vi "User_Login.vi"() -> ()   [LabVIEW 2019]
uses:
  <vilib>/Utility/file.llb/Read Delimited Spreadsheet (string).vi
  <vilib>/Utility/file.llb/Write Delimited Spreadsheet (string).vi
  <vilib>/Utility/file.llb/Write Delimited Spreadsheet (I64).vi
  <vilib>/numeric/Random Number (Range) U64.vi
panel:
  out "测试":bool
  in  "数组":u64[](array[numeric])
  in  "亮灯次数":i32=1
  in  "是否开始计时？":bool
  out "分数":i32
  out "难度":string="困难"
  out "闪烁间隔":i32=727
  out "超时时间":i32=500
  out "User name out":string
  out "时间到":bool
  out "字符串":string
  in  "选项卡控件":T1(tab)
  in  "密码":string
  in  "账号":string
  in  "登录界面_修改密码":bool
  in  "登陆界面_注册":bool
  in  "登录界面_登录":bool
  in  "登录界面_退出":bool
  in  "主界面_TOP10":bool
  in  "主界面_返回":bool
  in  "主界面_进入游戏":bool
  in  "主界面_游戏规则":bool
  in  "注册簇":T2
  in  "用户注册_注册":bool
  in  "用户注册_返回":bool
  in  "修改密码簇":T3
  in  "修改密码_返回":bool
  in  "修改密码_修改":bool
  in  "TOP10_返回":bool
  in  "游戏规则_返回":bool
  in  "读档":bool
  in  "存档":bool
  out "难度：分数":string
  out "倒计时":i32(slide) scale=-1.0..3635.0
  in  "User name in":string
  in  "结束":bool
  out "上":bool
  out "左":bool
  out "右":bool
  out "下":bool
  in  "OK":bool
  # "游戏开始时，第一次亮一\n个灯，然后我们需要点击一次已 \n，第二次会亮两个灯，包括第一\n次的灯，第三次亮三个，每次增\n加一个灯，你都需要按顺序点击\n，或者使用键盘的↑↓←→操作"
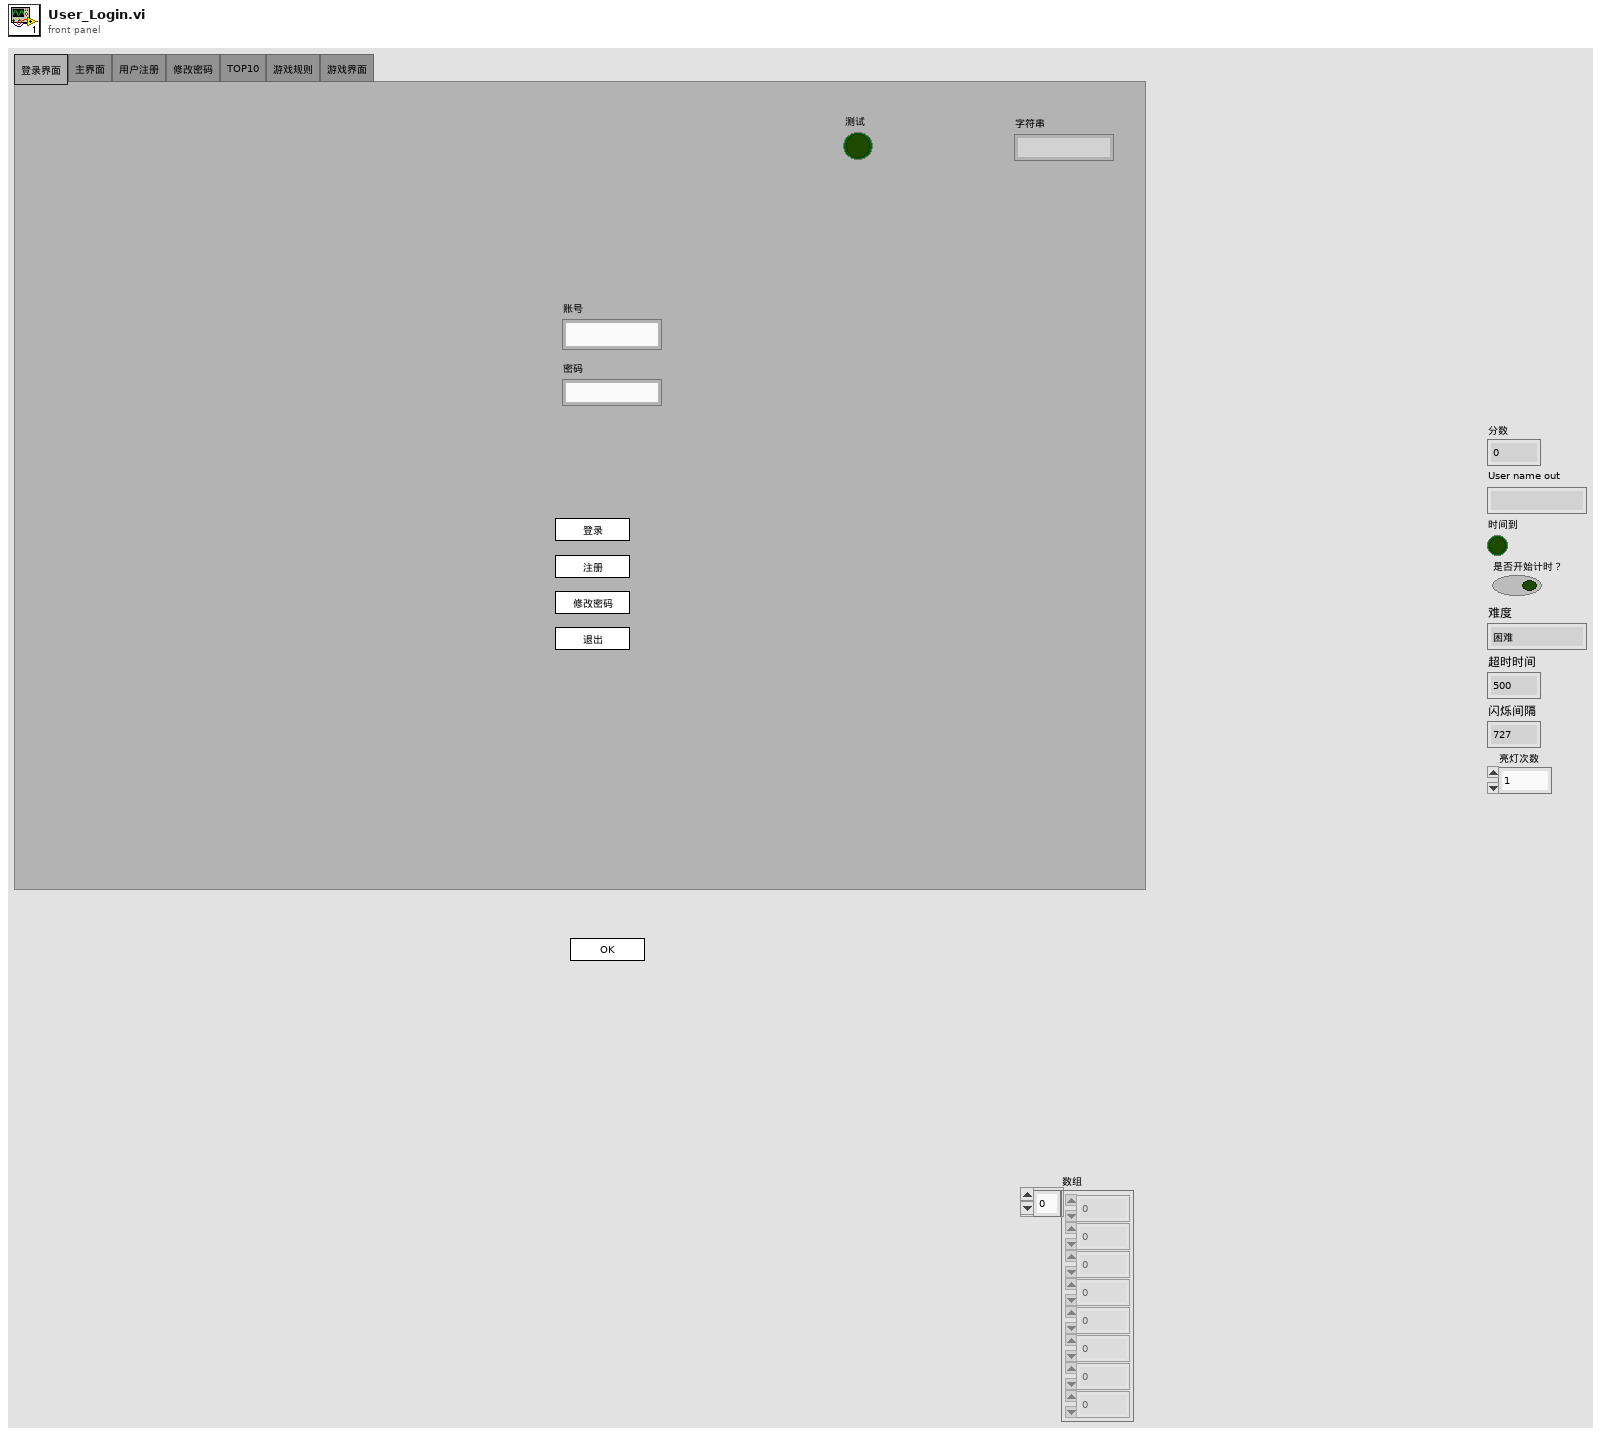
[diagram p1: front panel]
types:
  T1 = enum32{"登录界面", "主界面", "用户注册", "修改密码", "TOP10", "游戏规则", "游戏界面"}
  T2 = cluster{"注册账户":string, "注册密码":string, "确认密码":string}
  T3 = cluster{"账号":string, "旧密码":string, "新密码":string, "确认密码":string}
  T4 = typedef "选项卡枚举.ctl" = enum32{"登录界面", "主界面", "用户注册", "修改密码", "TOP10", "游戏规则", "游戏界面"}
  T5 = enum32{"Invalid", "Standard", "Closed", "Hidden", "Minimized", "Maximized"}
  T6 = enum32{"invalid app kind", "Development System", "Run Time System", "Student Edition", "Embedded LabVIEW", "Evaluation", "Custom"}
  T7 = typedef "按键枚举.ctl" = enum16{"读档", "存档", "按错", "退出", "黄", "红", "蓝", "绿"}
  T8 = cluster{"Core":cluster{"Current VI Reference":refnum<vi>, "Close Panel on Exit?":bool}, "Your Boolean data":bool, "注册账户":string, "注册密码":string, "修改密码_新密码":string, "修改密码_账户":string, "用户名":string, "难度_保存":string, "亮灯次数_保存":i32, "超时时间_保存":i32, "闪烁间隔_保存":i32, "积分_保存":i32}
  T9 = cluster{"Current VI Reference":refnum<vi>, "Close Panel on Exit?":bool}
  T10 = enum16{"Left Button", "Center Button", "Right Button", "Window Close"}
  T11 = typedef "eventvkey.ctl" = enum16{"ASCII", "Enter", "Return", "Shift", "Ctrl", "Alt", "Cmd", "Opt", "Caps", "NumLock", "Clear", "Break", "Up", "Down", "Left", "Right", "Insert", "Delete", "Home", "End", "PageUp", "PageDown", "Escape", "Help", "Pause", "ScrollLock", "F1", "F2", "F3", "F4", "F5", "F6", "F7", "F8", "F9", "F10", "F11", "F12", "F13", "F14", "F15", "F16", "F17", "F18", "F19", "F20", "F21", "F22", "F23", "F24", "Play", "VolumeUp", "VolumeDown", "Mute", "Two Byte Char"}
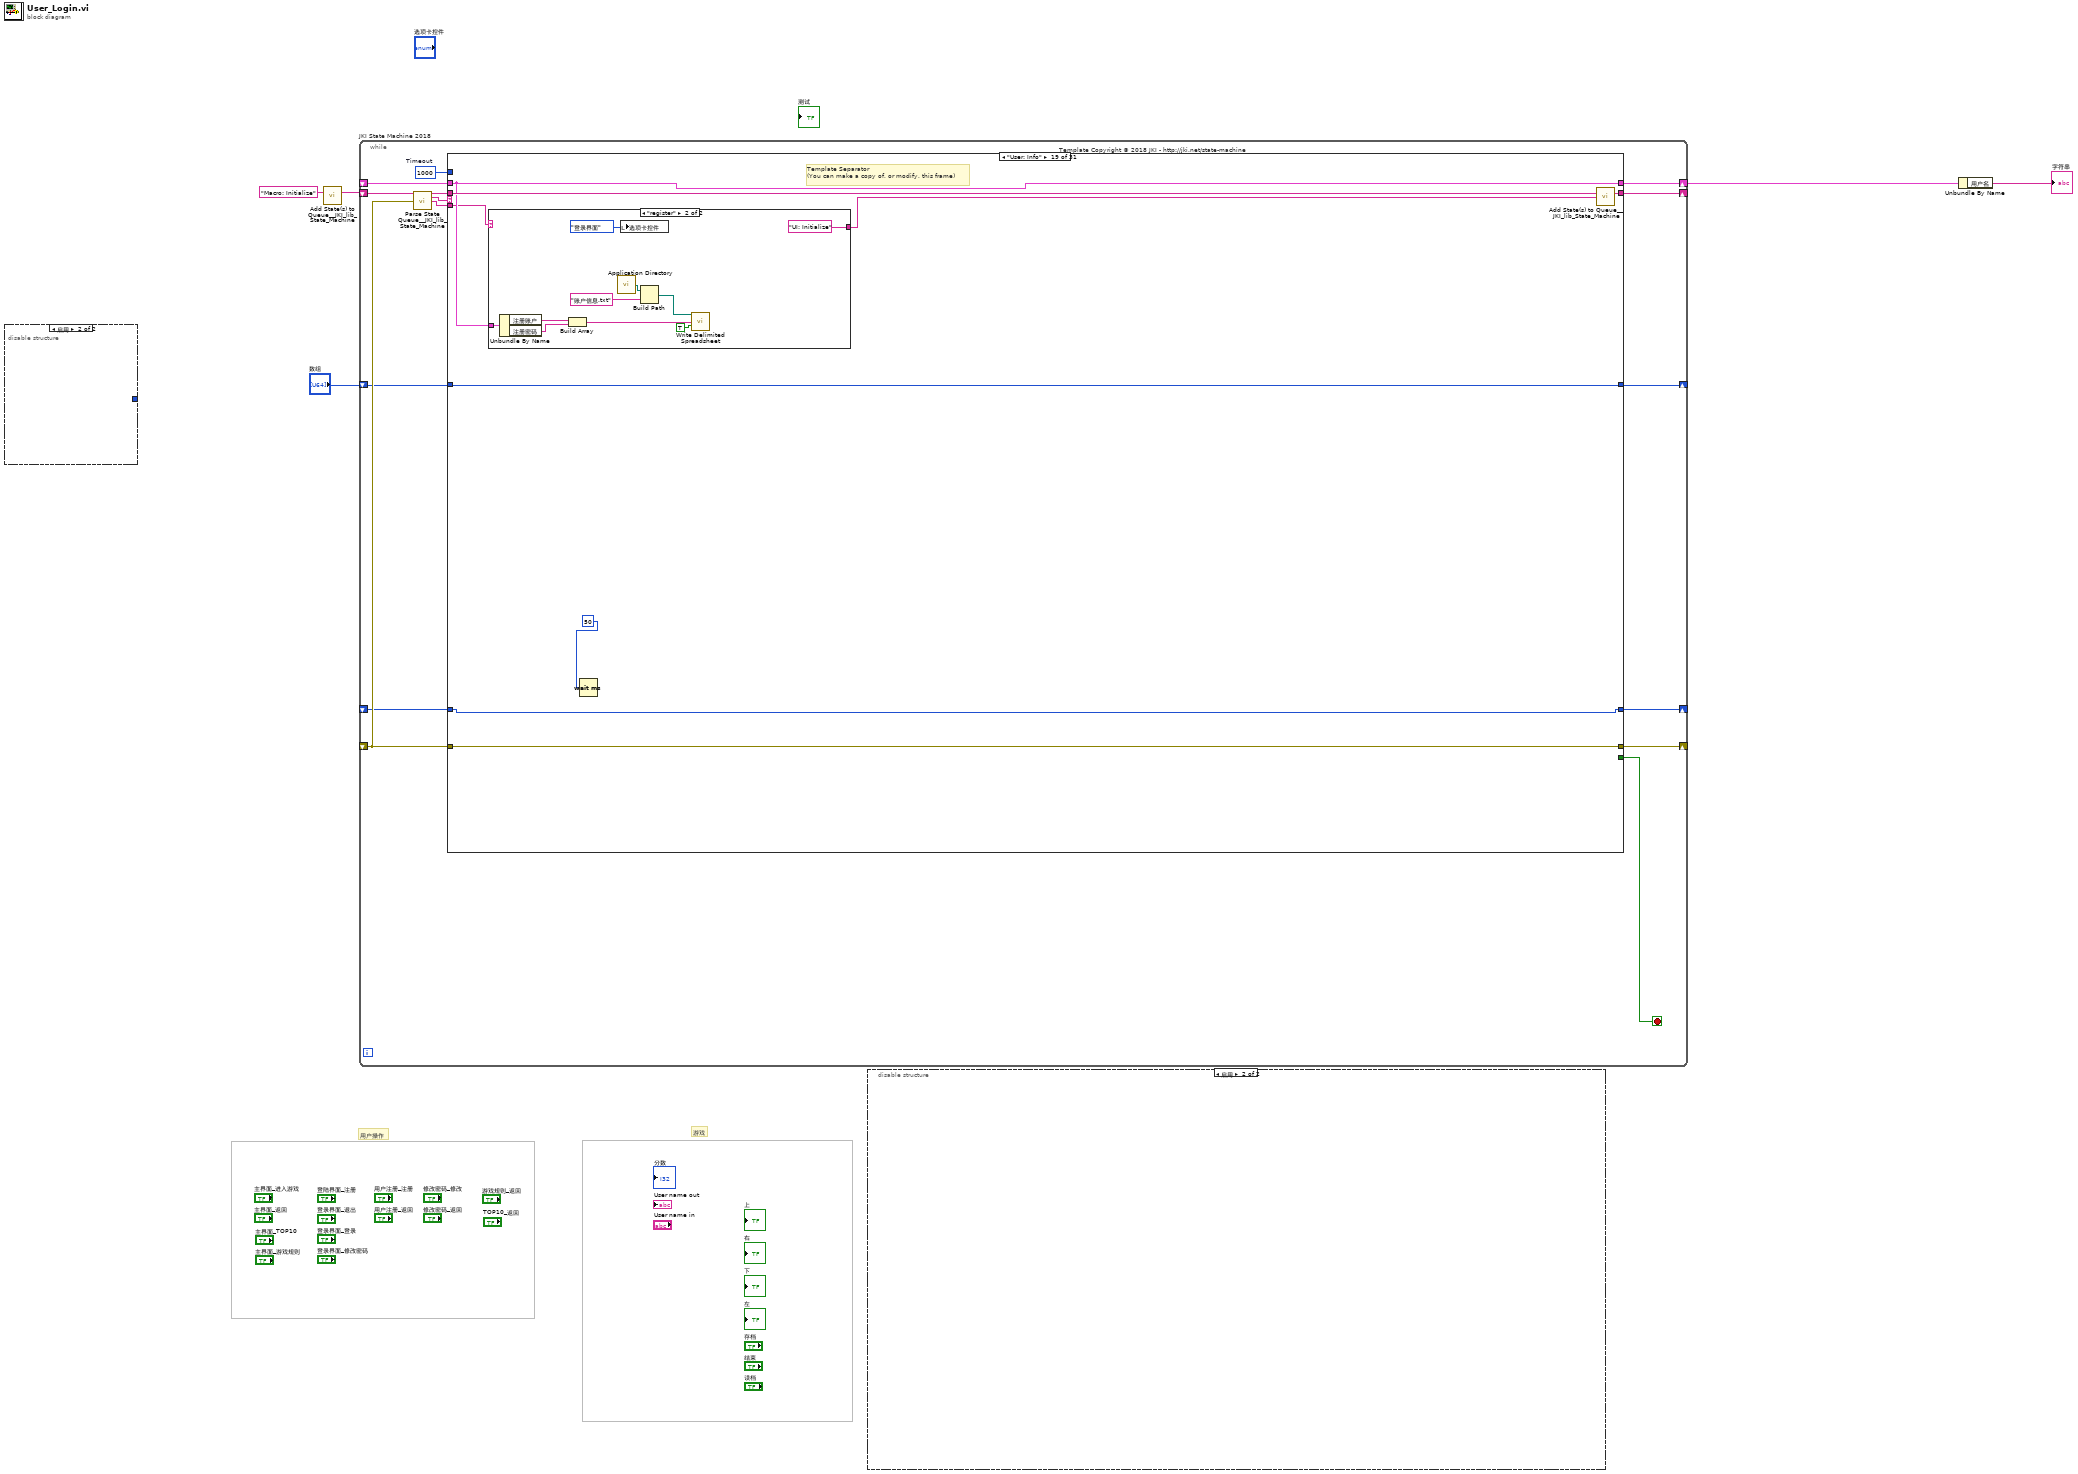
[diagram p0: block diagram]
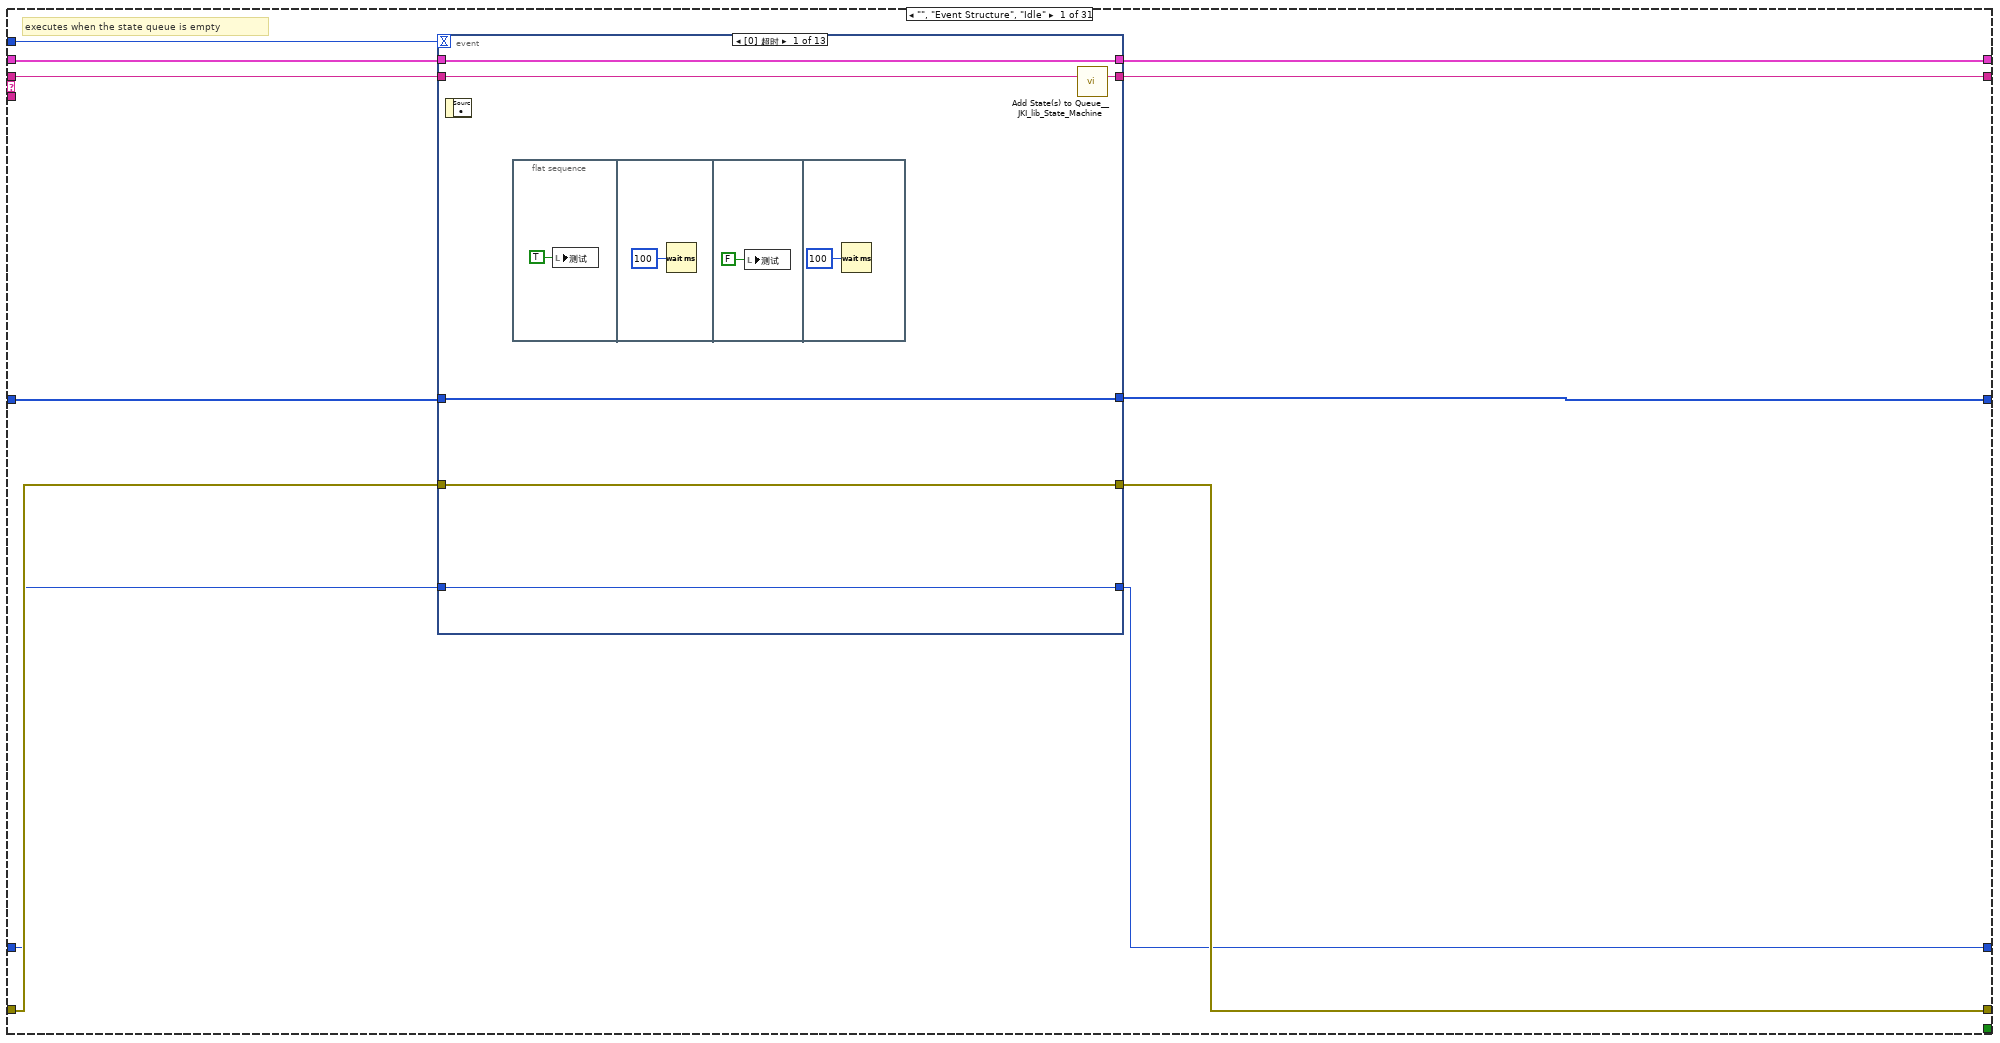
[diagram p2: hidden frame]
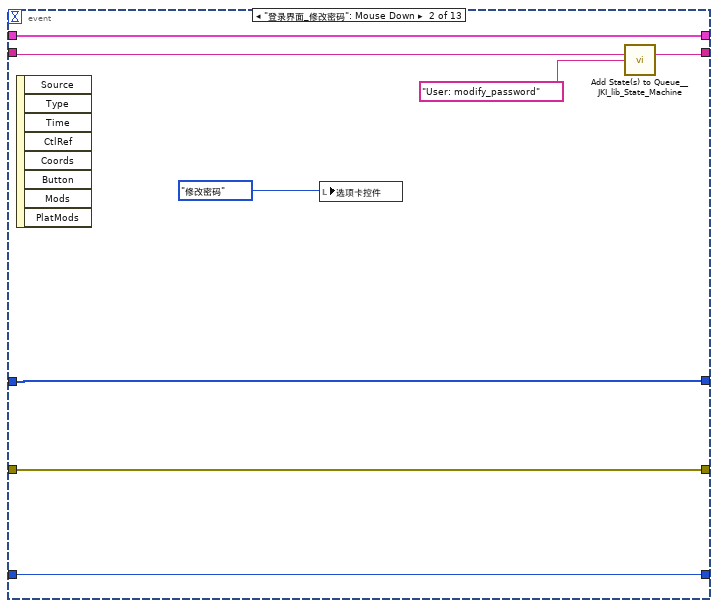
[diagram p3: hidden frame]
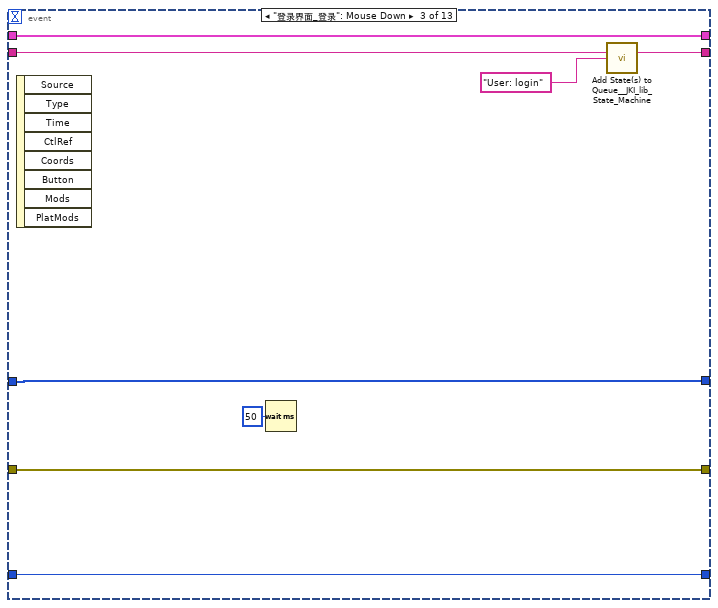
[diagram p4: hidden frame]
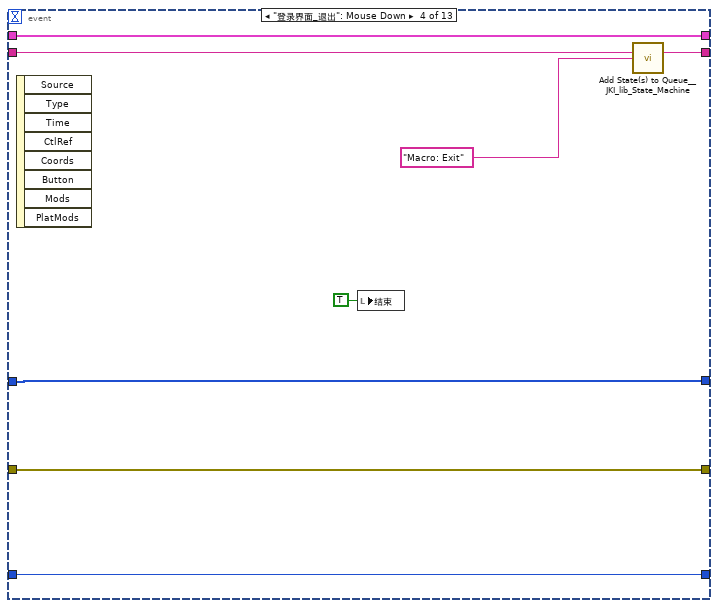
[diagram p5: hidden frame]
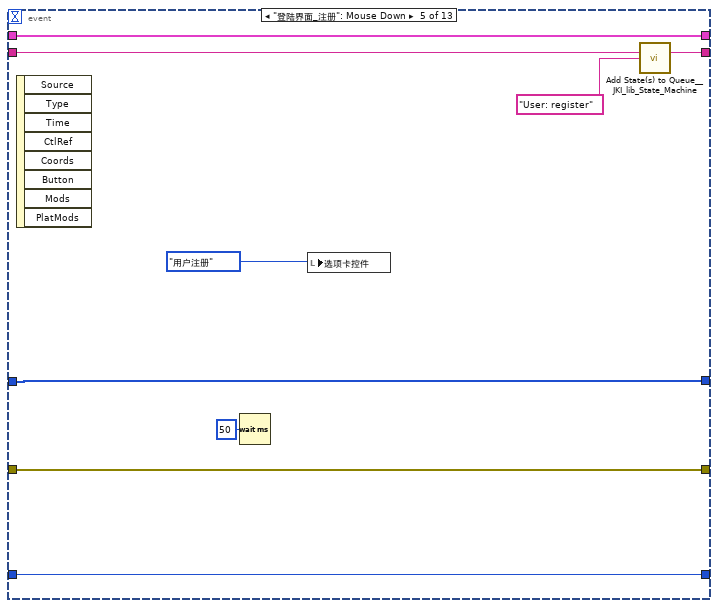
[diagram p6: hidden frame]
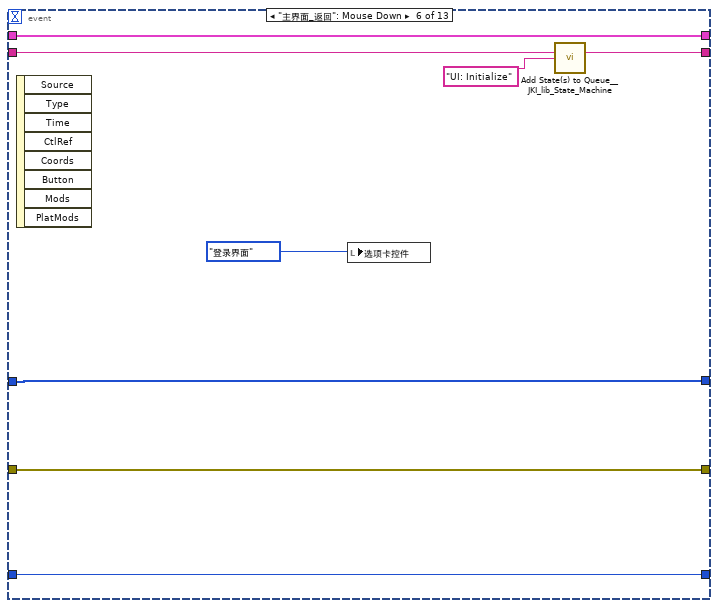
[diagram p7: hidden frame]
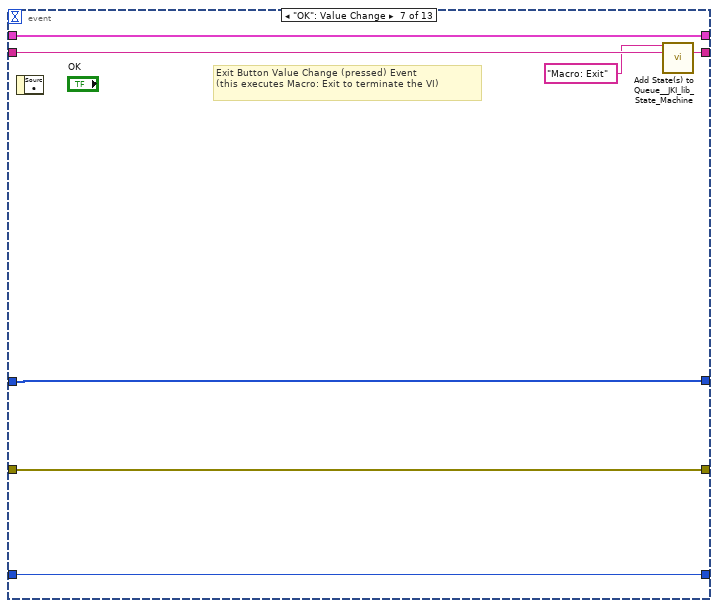
[diagram p8: hidden frame]
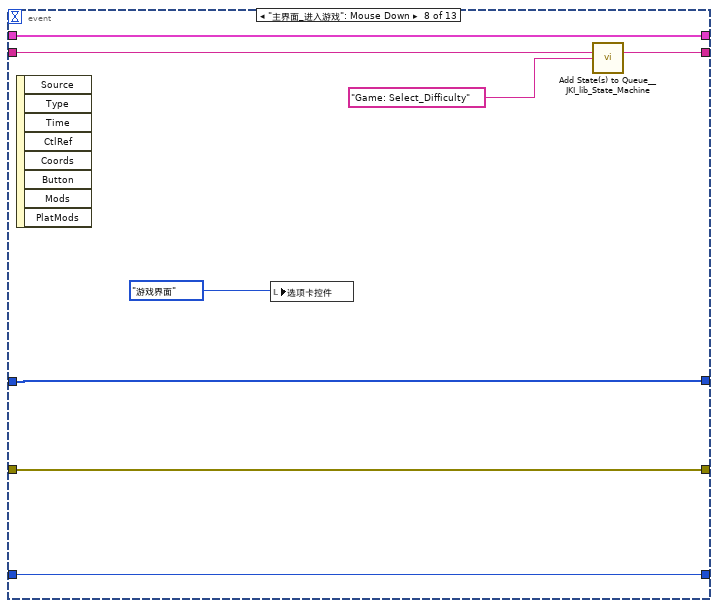
[diagram p9: hidden frame]
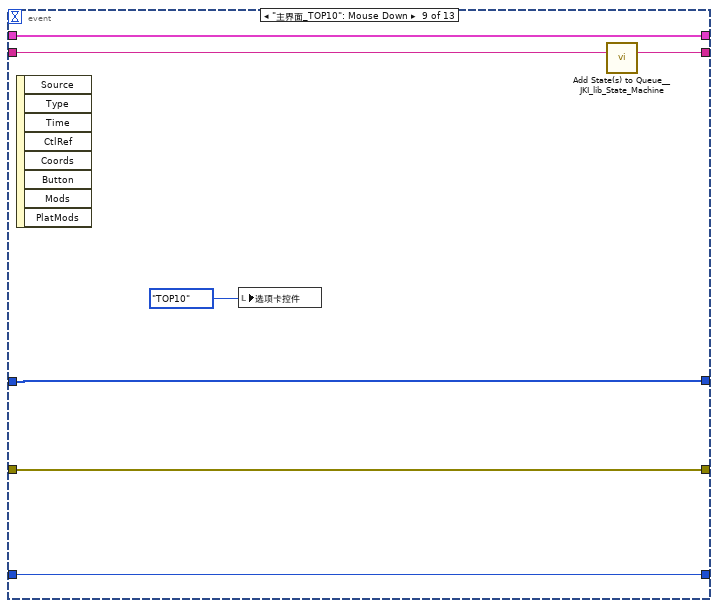
[diagram p10: hidden frame]
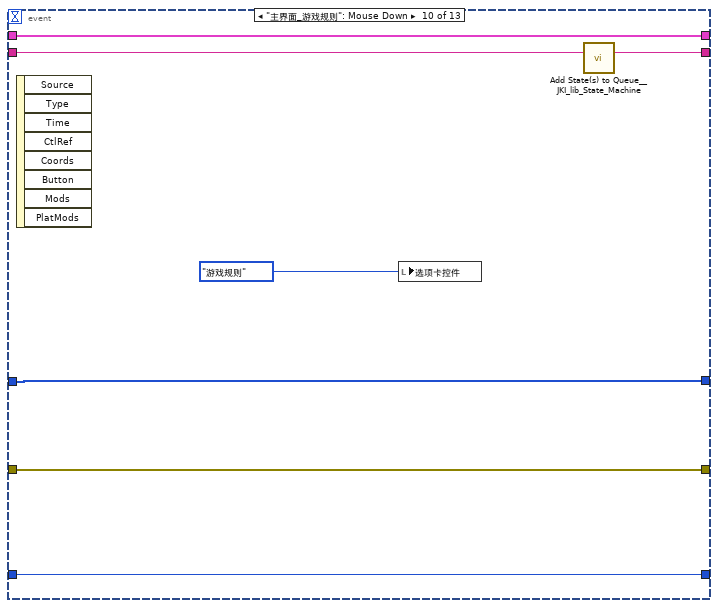
[diagram p11: hidden frame]
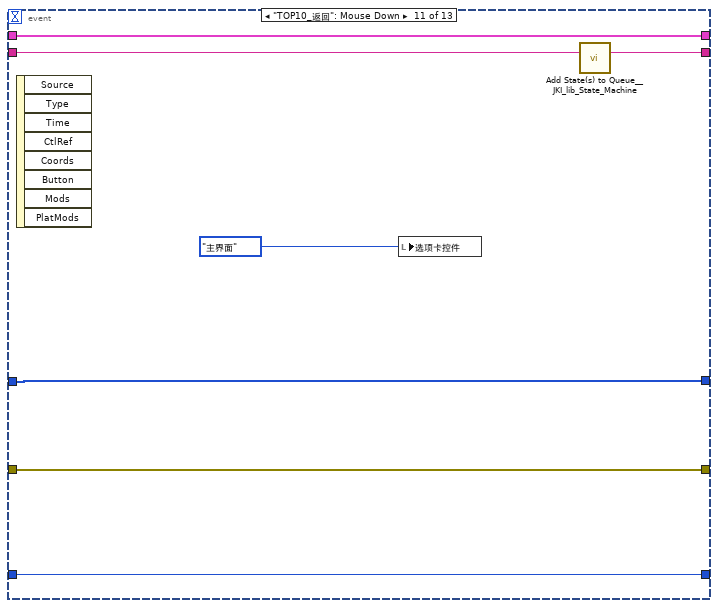
[diagram p12: hidden frame]
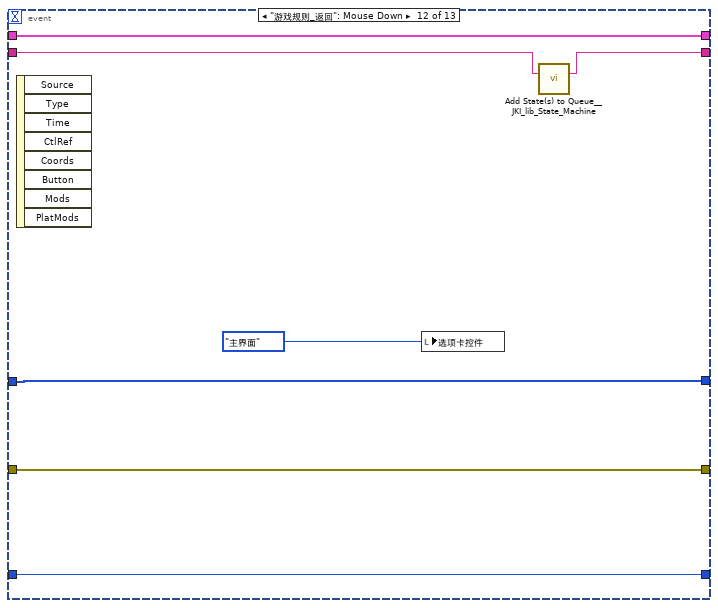
[diagram p13: hidden frame]
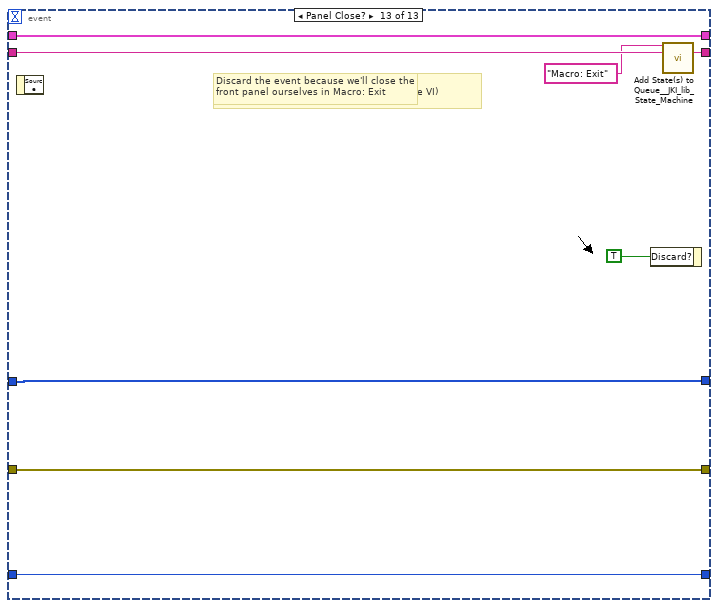
[diagram p14: hidden frame]
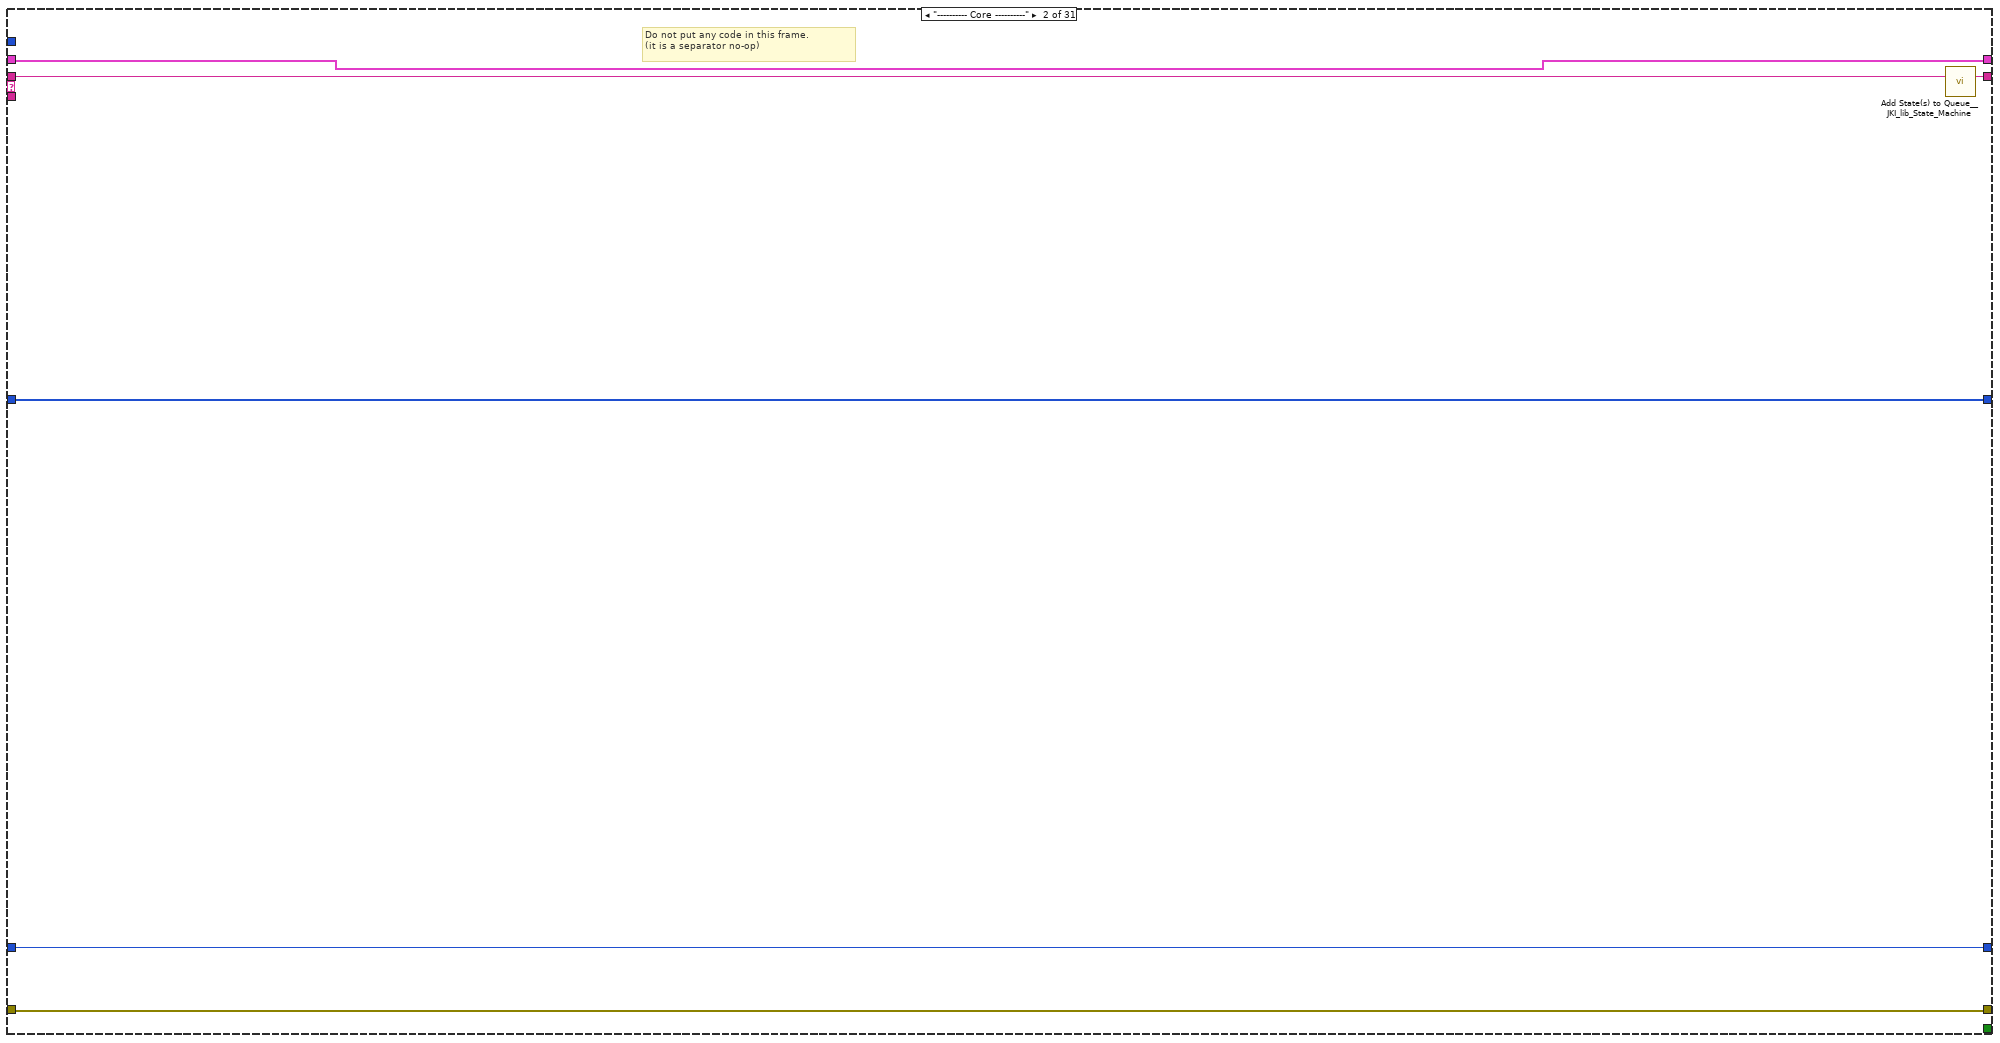
[diagram p15: hidden frame]
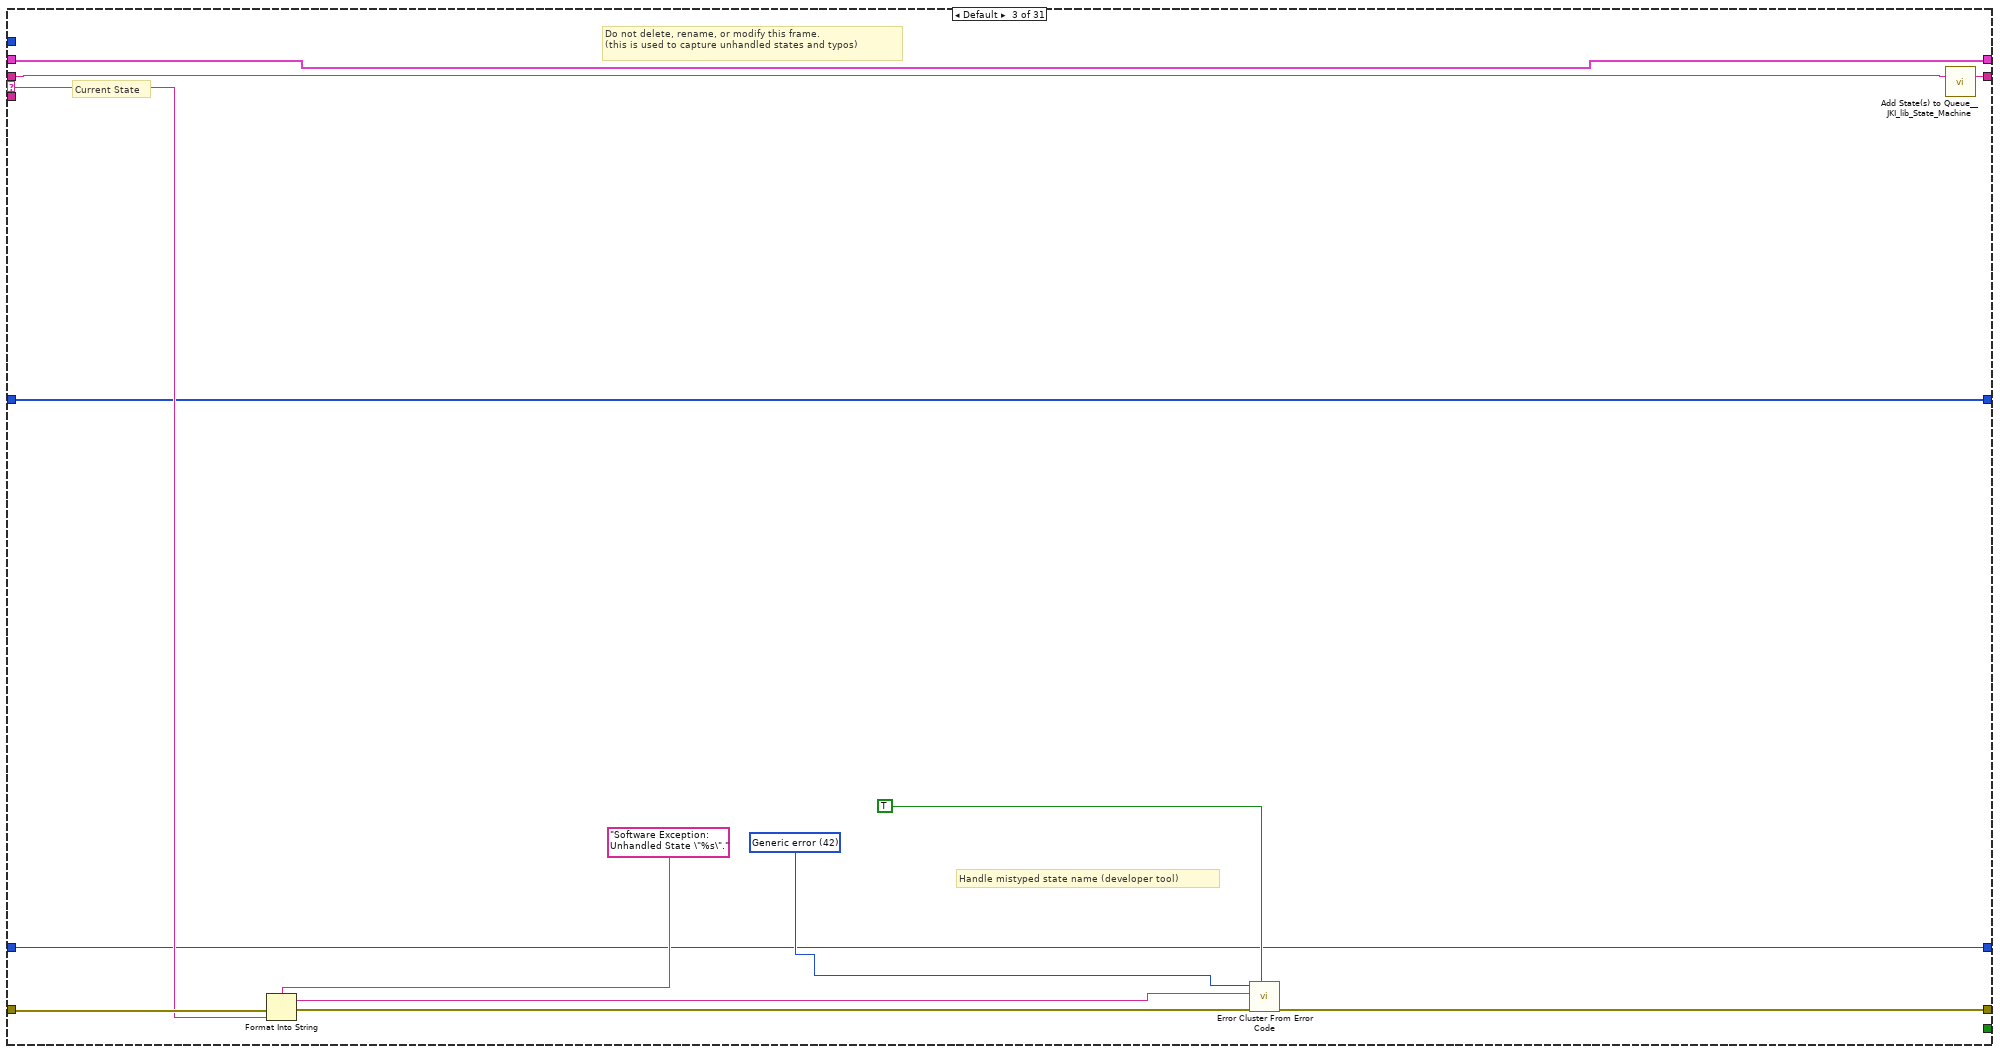
[diagram p16: hidden frame]
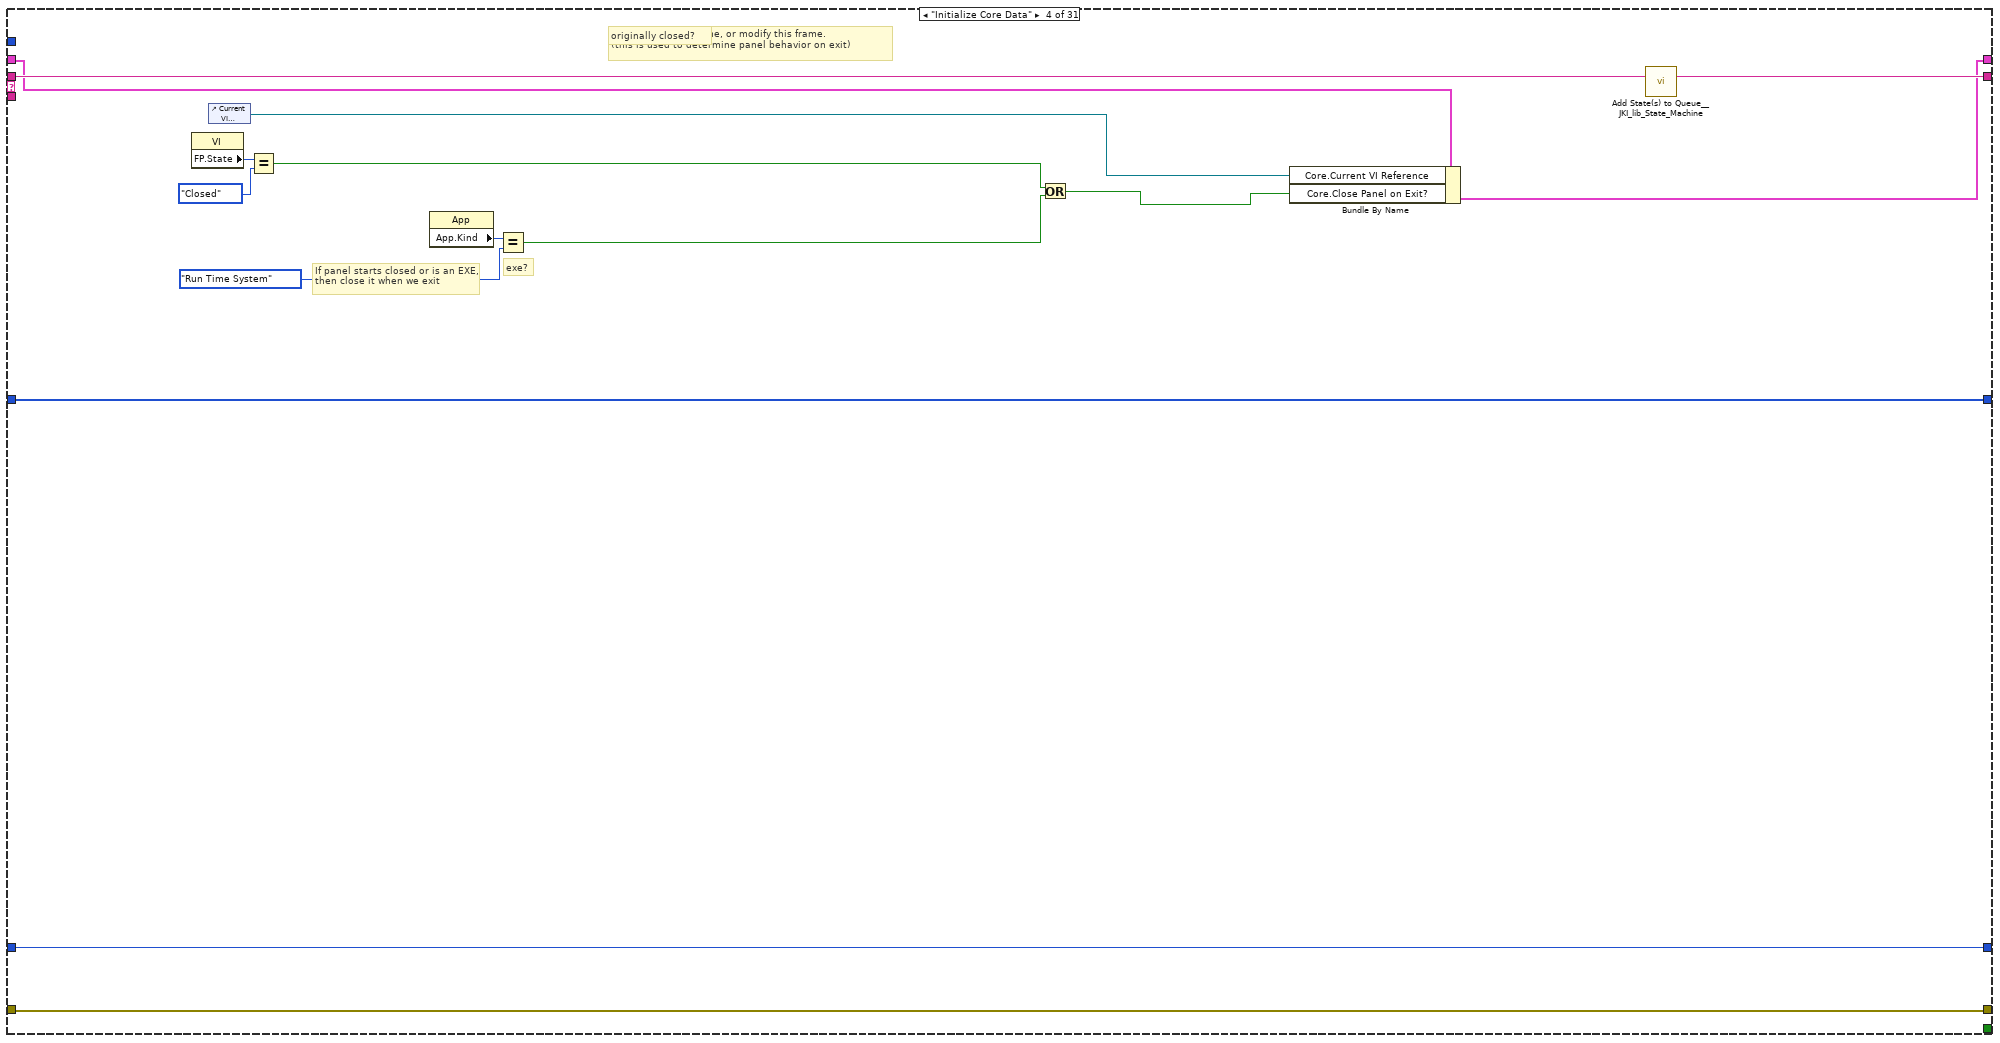
[diagram p17: hidden frame]
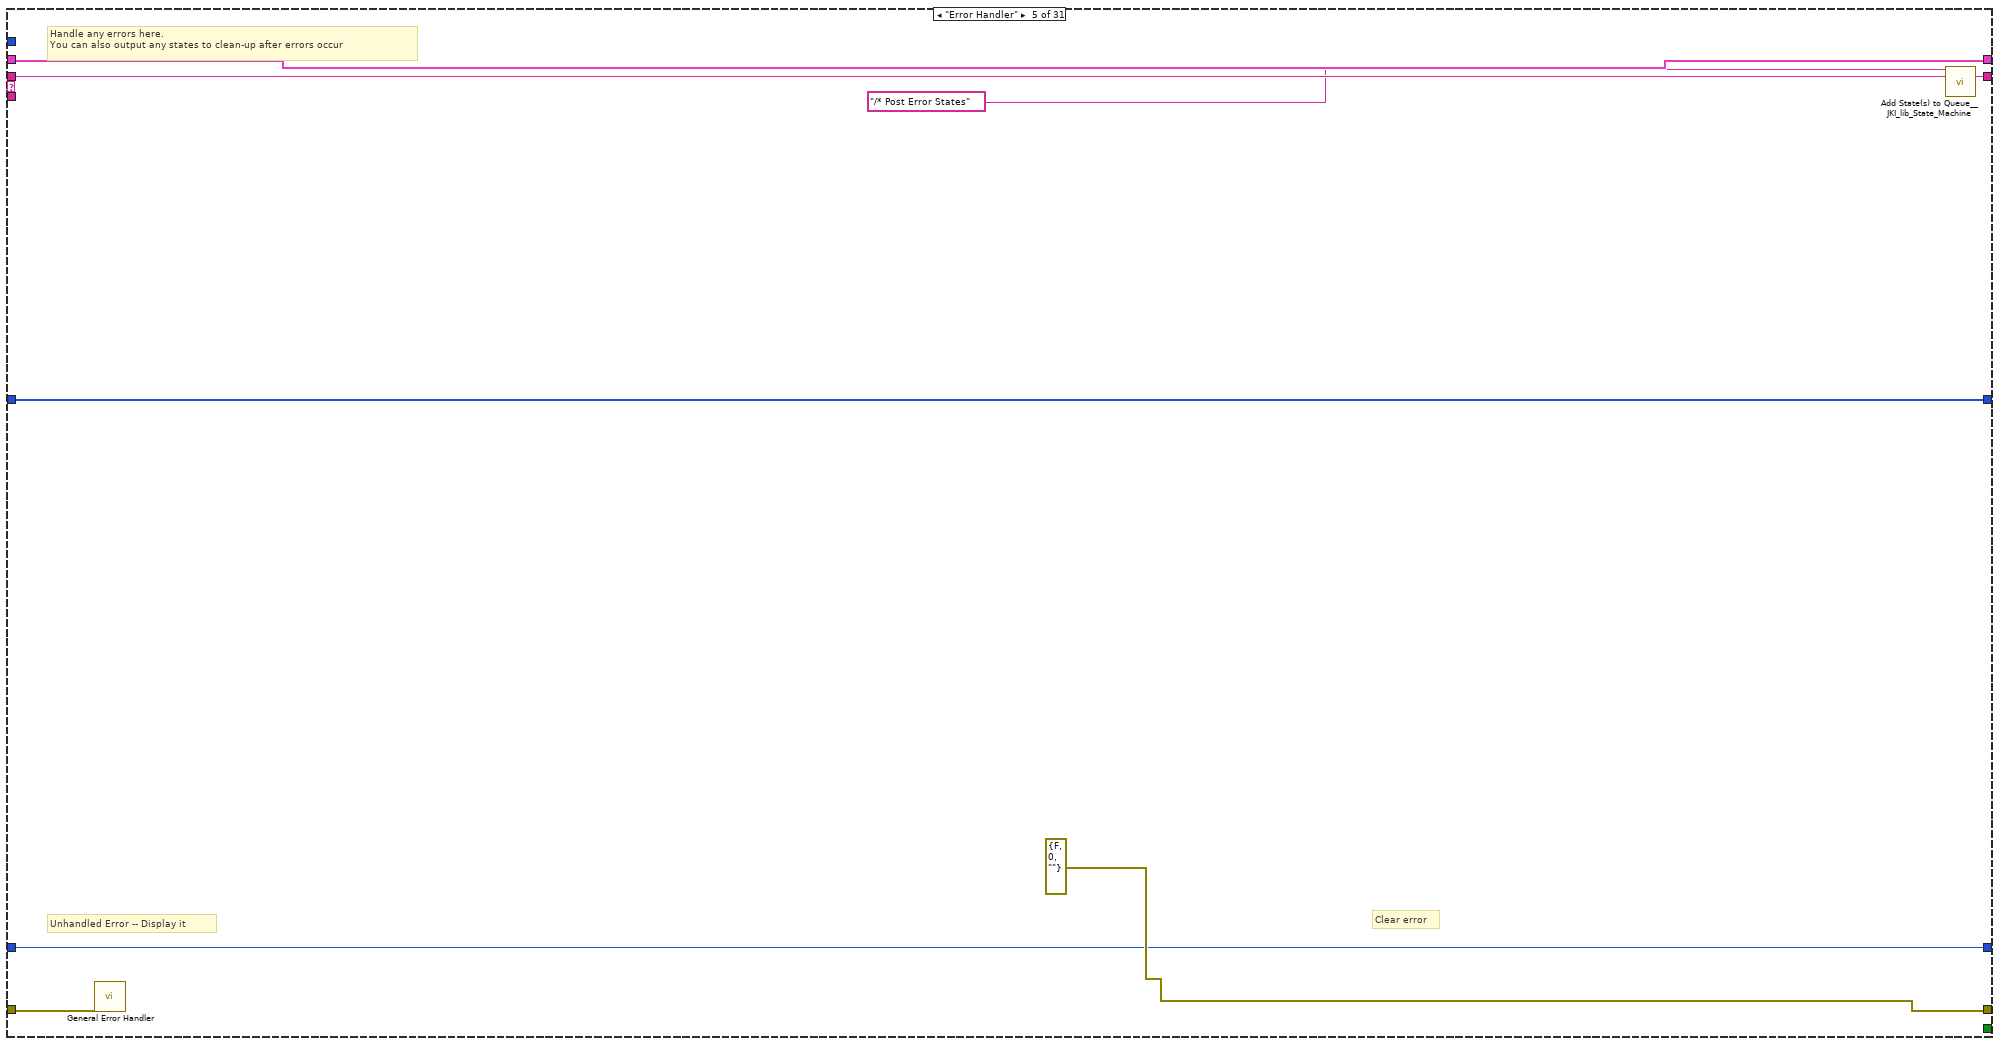
[diagram p18: hidden frame]
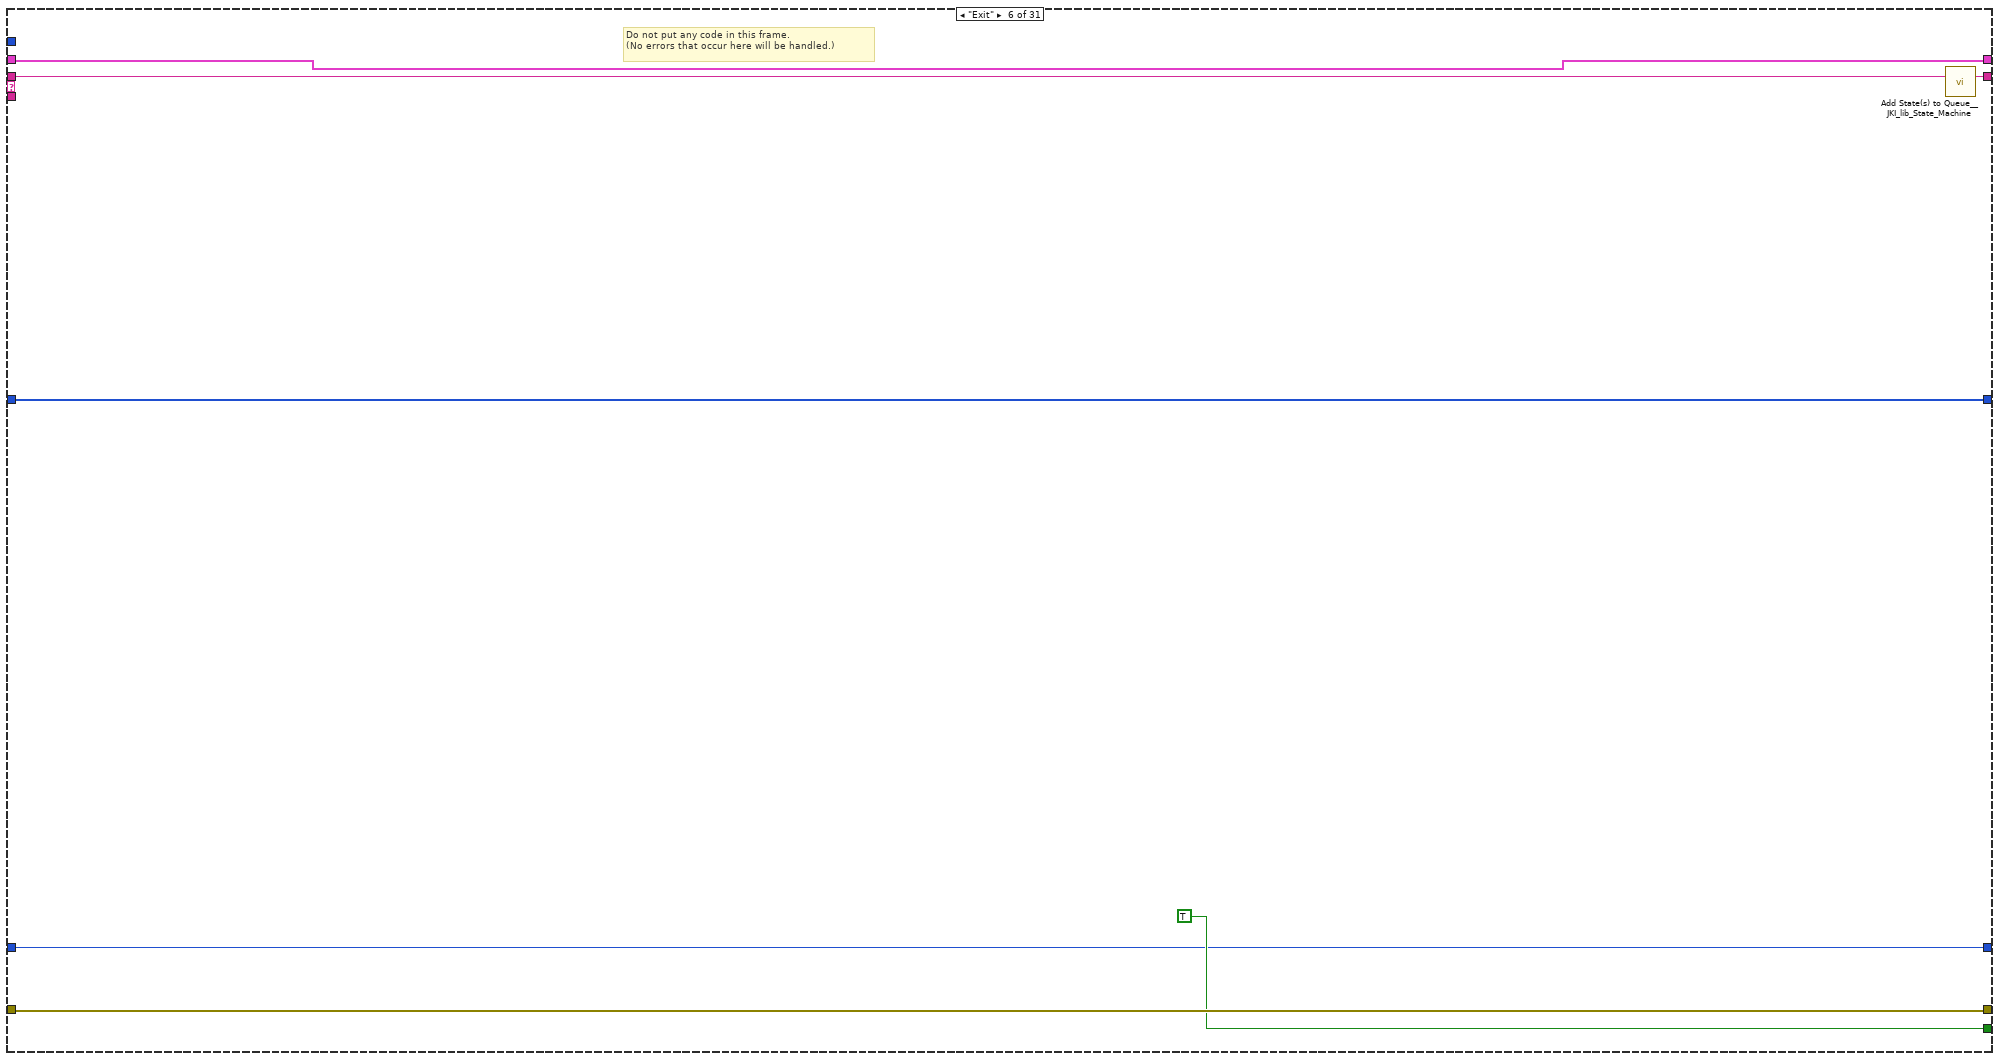
[diagram p19: hidden frame]
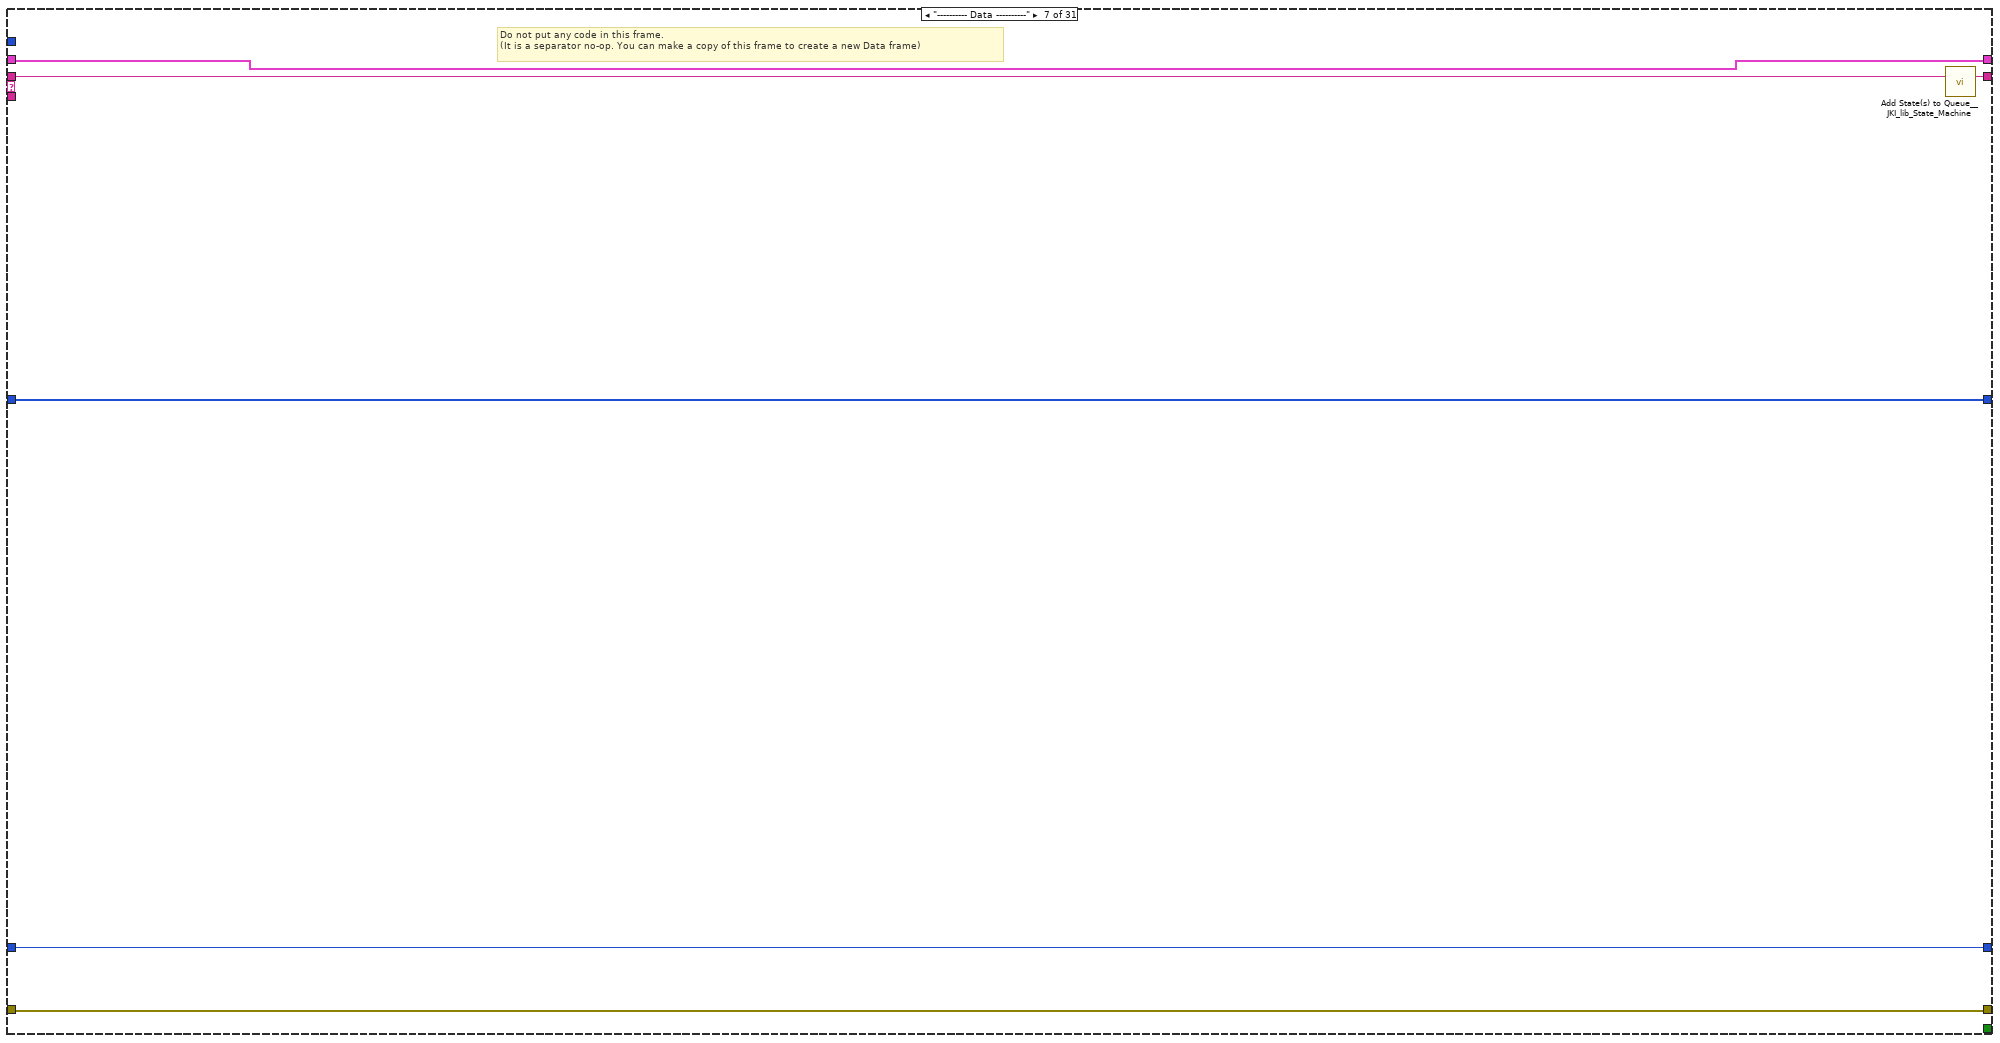
[diagram p20: hidden frame]
diagram:
  # "游戏"
  # "用户操作"
  n1 = disable-structure shown="启用" {
    disable-tunnel: [w6 _] -> _
    frame Disabled {
      n2 = for {
        N: 50 -> [_]
        tunnel: [w8] -> w6 mode=indexing
        # "生成50个随机数"
        n3 = call-poly <vilib>:"Random Number (Range).vi"("lower bound (0)"=u64 0, "upper bound (100)"=u64 3) -> ("number"=w8:u64)  [unwired: 9 in]
      }
    }
    frame Enabled {
    }
  }
  n4 = call <vilib>:"Add State(s) to Queue__JKI_lib_State_Machine.vi"("State(s) in (\"\")"="Macro: Initialize") -> ("States Out"=w5:string)  [unwired: 14 in]
  n5 = while "JKI State Machine 2018" {
    shift-right: [w18] -> w3
    shift-left: _ -> [w17]
    shift-right: [w21] -> _
    shift-left: _ -> [w15]
    shift-right: [w20] -> _
    shift-left: w5 -> [w22]
    shift-right: [w13] -> _
    shift-left: "数组" -> [w14]
    shift-right: [w12] -> _
    shift-left: _ -> [w11]
    stop <- w19 stop-if-true
    w16 = 1000  # Timeout
    # "Template Copyright © 2018 JKI - http://jki.net/state-machine"
    n6 = call <vilib>:"Parse State Queue__JKI_lib_State_Machine.vi"("State Queue"=w22, "Error In (no error)"=w15) -> ("Remaining States"=w24:string, "Current State"=w25:string, "Arguments"=w23:string)  [unwired: 11 in]
    n7 = case shown="\"User: Info\"" w25 {
      selector: w25 -> [_ _ w147 _ _ _ _ _ _ _ _ _ _ _ _ _ _ _ _ _ _ _ _ _ _ _ _ _ _ _ _]
      tunnel: w24 -> [w36 w144 w151 w172 w180 w187 w193 w211 w219 w225 w231 w239 w252 w323 w330 w342 w348 w357 w447 w483 w569 w601 w607 w627 w646 w672 w690 w824 w845 w862 w871]
      tunnel: w23 -> [_ _ _ _ _ _ _ _ _ _ _ w234 w246 _ _ _ _ _ w441 _ _ _ _ _ _ _ _ _ _ _ _]
      tunnel: w17 -> [w34 w141 w149 w165 w177 w185 w190 _ w214 w222 w229 w237 w248 w320 w327 w339 w345 w353 w444 w479 w547 w598 w604 w615 w643 w669 w687 w821 w833 w859 w868]
      tunnel: [w33 w142 w153 w169 errorcluster {"status"=FALSE, "code"=0, "source"=""} ("error out") w184 w191 w208 w215 w223 w228 w235 w249 w321 w328 w340 w346 w355 w445 w481 w567 w599 w605 w625 w644 w670 w688 w822 w843 w860 w869] -> w21
      tunnel: w15 -> [w32 w142 w152 w169 w176 w184 w191 w208 w216 w223 w228 w236 w250 w321 w328 w340 w346 w355 w445 w481 w567 w599 w605 w625 w644 w670 w688 w822 w843 w860 w869]
      tunnel: [w35 w143 w150 w171 w179 w186 w192 w210 w218 w224 w230 w238 w251 w322 w329 w341 w347 w356 w446 w482 w568 w600 w606 w626 w645 w671 w689 w823 w844 w861 w870] -> w20
      tunnel: [_ _ _ _ _ TRUE _ _ _ _ _ _ _ _ _ _ _ _ _ _ _ _ _ _ _ _ _ _ _ _ _] -> w19
      tunnel: [w31 w141 w149 w170 w177 w185 w190 w209 w214 w222 w229 w237 w248 w320 w327 w339 w345 w352 w444 w478 w546 w598 w604 w614 w643 w669 w687 w821 w830 w859 w868] -> w18
      tunnel: w16 -> [w30 _ _ _ _ _ _ _ _ _ _ _ _ _ _ _ _ _ _ _ _ _ _ _ _ _ _ _ _ _ _]
      tunnel: w14 -> [w29 w140 w146 w159 w173 w182 w189 w195 w213 w221 w227 w233 w245 w319 w325 w332 w344 w349 w440 w476 w544 w597 w603 w609 w641 w668 w684 w812 w827 w848 w867]
      tunnel: [w28 w140 w146 w159 w173 w182 w189 w195 w213 w221 w227 w233 w245 w319 w325 w332 w344 w349 w440 w476 w544 w597 w603 w609 w641 w668 w684 w812 w827 w848 w867] -> w13
      tunnel: [w26 w139 w145 w158 w174 w181 w188 0 w212 w220 w226 w232 w244 w318 w324 w331 w343 w350 w439 w475 w545 w596 w602 w608 w638 1 w677 w811 w828 w846 w866] -> w12
      tunnel: w11 -> [w27 w139 w145 w158 w174 w181 w188 _ w212 w220 w226 w232 w244 w318 w324 w331 w343 w350 w439 w475 w545 w596 w602 w608 w638 _ w685 w811 w828 w846 w866]
      frame "", "Event Structure", "Idle" {
        # "executes when the state queue is empty"
        n8 = event shown="[0] 超时" {
          selector: _ -> [_ _ _ _ _ _ _ _ _ _ _ _ _]
          dyn-events: _ -> [_ _ _ _ _ _ _ _ _ _ _ _ _]
          timeout: w30 -> [_ _ _ _ _ _ _ _ _ _ _ _ _]
          tunnel: w36 -> [w42 w52 w60 w67 w77 w84 w94 w100 w106 w115 w122 w128 w138]
          tunnel: [w41 w53 w61 w68 w78 w85 w93 w99 w107 w114 w121 w129 w137] -> w35
          tunnel: w34 -> [w39 w54 w62 w70 w79 w87 w91 w102 w108 w116 w123 w127 w135]
          tunnel: [w40 w50 w58 w69 w75 w86 w92 w101 w109 w112 w119 w126 w136] -> w33
          tunnel: w32 -> [w40 w50 w58 w69 w75 w86 w92 w101 w109 w112 w119 w126 w136]
          tunnel: [w39 w54 w62 w70 w79 w87 w91 w102 w108 w116 w123 w127 w135] -> w31
          tunnel: w29 -> [w38 w48 w56 w64 w72 w81 w89 w96 w104 w111 w118 w125 w132]
          tunnel: [w38 w48 w56 w64 w72 w81 w89 w96 w104 w111 w118 w125 w132] -> w28
          tunnel: w27 -> [w37 w47 w55 w63 w71 w80 w88 w95 w103 w110 w117 w124 w131]
          tunnel: [w37 w47 w55 w63 w71 w80 w88 w95 w103 w110 w117 w124 w131] -> w26
          event Timeout {
            n9 = event-data() -> ()  [unwired: 1 in, 1 out]
            n10 = flat-sequence {
              frame #0 {
                n11 = local write "测试"(TRUE ("测试")) -> ()
              }
              frame #1 {
                n12 = Wait (ms)(milliseconds to wait=u32 100 ("等待时间（毫秒）")) -> ()  [unwired: 1 out]
              }
              frame #2 {
                n13 = local write "测试"(FALSE ("测试")) -> ()
              }
              frame #3 {
                n14 = Wait (ms)(milliseconds to wait=u32 100 ("等待时间（毫秒）")) -> ()  [unwired: 1 out]
              }
            }
            n15 = call <vilib>:"Add State(s) to Queue__JKI_lib_State_Machine.vi"("State(s) in (\"\")"=w42) -> ("States Out"=w41:string)  [unwired: 14 in]
          }
          event "登录界面_修改密码": Mouse Down {
            n16 = event-data() -> ()  [unwired: 1 in, 8 out]
            n17 = local write "选项卡控件"(选项卡枚举."修改密码" ("枚举")) -> ()
            n18 = call <vilib>:"Add State(s) to Queue__JKI_lib_State_Machine.vi"("State(s) in (\"\")"=w52, "State(s) at Back (\"\")"="User: modify_password" ("State(s) at Back (\"\")")) -> ("States Out"=w53:string)  [unwired: 13 in]
          }
          event "登录界面_登录": Mouse Down {
            n19 = event-data() -> ()  [unwired: 1 in, 8 out]
            n20 = Wait (ms)(milliseconds to wait=u32 50 ("等待时间（毫秒）")) -> ()  [unwired: 1 out]
            n21 = call <vilib>:"Add State(s) to Queue__JKI_lib_State_Machine.vi"("State(s) in (\"\")"=w60, "State(s) at Back (\"\")"="User: login" ("State(s) at Back (\"\")")) -> ("States Out"=w61:string)  [unwired: 13 in]
          }
          event "登录界面_退出": Mouse Down {
            n22 = event-data() -> ()  [unwired: 1 in, 8 out]
            n23 = local write "结束"(TRUE ("结束")) -> ()
            n24 = call <vilib>:"Add State(s) to Queue__JKI_lib_State_Machine.vi"("State(s) in (\"\")"=w67, "State(s) at Back (\"\")"="Macro: Exit") -> ("States Out"=w68:string)  [unwired: 13 in]
          }
          event "登陆界面_注册": Mouse Down {
            n25 = event-data() -> ()  [unwired: 1 in, 8 out]
            n26 = Wait (ms)(milliseconds to wait=u32 50 ("等待时间（毫秒）")) -> ()  [unwired: 1 out]
            n27 = local write "选项卡控件"(选项卡枚举."用户注册" ("枚举")) -> ()
            n28 = call <vilib>:"Add State(s) to Queue__JKI_lib_State_Machine.vi"("State(s) in (\"\")"=w77, "State(s) at Back (\"\")"="User: register" ("State(s) at Back (\"\")")) -> ("States Out"=w78:string)  [unwired: 13 in]
          }
          event "主界面_返回": Mouse Down {
            n29 = event-data() -> ()  [unwired: 1 in, 8 out]
            n30 = local write "选项卡控件"(选项卡枚举."登录界面" ("枚举")) -> ()
            n31 = call <vilib>:"Add State(s) to Queue__JKI_lib_State_Machine.vi"("State(s) in (\"\")"=w84, "State(s) at Back (\"\")"="UI: Initialize") -> ("States Out"=w85:string)  [unwired: 13 in]
          }
          event "OK": Value Change {
            # "Exit Button Value Change (pressed) Event\n(this executes Macro: Exit to terminate the VI)"
            n32 = event-data() -> ()  [unwired: 1 in, 1 out]
            n33 = call <vilib>:"Add State(s) to Queue__JKI_lib_State_Machine.vi"("State(s) in Front (\"\")"="Macro: Exit", "State(s) in (\"\")"=w94) -> ("States Out"=w93:string)  [unwired: 13 in]
          }
          event "主界面_进入游戏": Mouse Down {
            n34 = event-data() -> ()  [unwired: 1 in, 8 out]
            n35 = local write "选项卡控件"(选项卡枚举."游戏界面" ("枚举")) -> ()
            n36 = call <vilib>:"Add State(s) to Queue__JKI_lib_State_Machine.vi"("State(s) in (\"\")"=w100, "State(s) at Back (\"\")"="Game: Select_Difficulty") -> ("States Out"=w99:string)  [unwired: 13 in]
          }
          event "主界面_TOP10": Mouse Down {
            n37 = event-data() -> ()  [unwired: 1 in, 8 out]
            n38 = local write "选项卡控件"(选项卡枚举."TOP10" ("枚举")) -> ()
            n39 = call <vilib>:"Add State(s) to Queue__JKI_lib_State_Machine.vi"("State(s) in (\"\")"=w106) -> ("States Out"=w107:string)  [unwired: 14 in]
          }
          event "主界面_游戏规则": Mouse Down {
            n40 = event-data() -> ()  [unwired: 1 in, 8 out]
            n41 = local write "选项卡控件"(选项卡枚举."游戏规则" ("枚举")) -> ()
            n42 = call <vilib>:"Add State(s) to Queue__JKI_lib_State_Machine.vi"("State(s) in (\"\")"=w115) -> ("States Out"=w114:string)  [unwired: 14 in]
          }
          event "TOP10_返回": Mouse Down {
            n43 = event-data() -> ()  [unwired: 1 in, 8 out]
            n44 = local write "选项卡控件"(选项卡枚举."主界面" ("枚举")) -> ()
            n45 = call <vilib>:"Add State(s) to Queue__JKI_lib_State_Machine.vi"("State(s) in (\"\")"=w122) -> ("States Out"=w121:string)  [unwired: 14 in]
          }
          event "游戏规则_返回": Mouse Down {
            n46 = event-data() -> ()  [unwired: 1 in, 8 out]
            n47 = local write "选项卡控件"(选项卡枚举."主界面" ("枚举")) -> ()
            n48 = call <vilib>:"Add State(s) to Queue__JKI_lib_State_Machine.vi"("State(s) in (\"\")"=w128) -> ("States Out"=w129:string)  [unwired: 14 in]
          }
          event Panel Close? {
            # "Discard the event because we'll close the front panel ourselves in Macro: Exit"
            # "Close Panel button (pressed) Event\n(this executes Macro: Exit to terminate the VI)"
            n49 = event-data() -> ()  [unwired: 1 in, 1 out]
            n50 = event-data("Discard?"=TRUE) -> ()  [unwired: 1 in, 1 out]
            n51 = call <vilib>:"Add State(s) to Queue__JKI_lib_State_Machine.vi"("State(s) in Front (\"\")"="Macro: Exit", "State(s) in (\"\")"=w138) -> ("States Out"=w137:string)  [unwired: 13 in]
          }
        }
      }
      frame "---------- Core ----------" {
        # "Do not put any code in this frame.\n(it is a separator no-op)"
        n52 = call <vilib>:"Add State(s) to Queue__JKI_lib_State_Machine.vi"("State(s) in (\"\")"=w144) -> ("States Out"=w143:string)  [unwired: 14 in]
      }
      frame Default {
        w156 = 42 items=["No error", "Argument error", "Memory is full", "Out of zone", "End of file", "File already open", "Generic file I/O error", "File not found", "File permission error", "Disk is full", "Duplicate path", "Too many files open", "System feature not enabled", "Resource file not found", "Cannot add resource", "Resource not found", "Image not found", "Image memory error", "Pen does not exist", "Config type invalid", "Config token not found", "Config parse error", "Config memory error", "Bad external code format", "Bad external code offset", "External code not present", "Null window", "Destroy window error", "Null menu", "Print aborted", "Bad print record", "Print driver error", "Windows error during printing", "Memory error during printing", "Print dialog error", "Generic print error", "Invalid device refnum", "Device not found", "Device parameter error", "Device unit error", "Cannot open device", "Device call aborted", "Generic error", "Cancelled by user", "Object ID too low", "Object ID too high", "Object not in heap", "Unknown heap", "Unknown object (invalid DefProc)", "Unknown object (DefProc not in table)", "Message out of range", "Invalid (null) method", "Unknown message", "Manager call not supported", "Bad address", "Network operation in progress", "Network operation timed out", "Connection is busy", "Network attribute not supported", "Network error", "Address in use", "System out of memory", "Connection aborted", "Connection refused", "Not connected", "Already connected", "Connection closed", "Initialization error (interapplication manager)", "Bad occurrence", "Wait on unbound occurrence handler", "Occurrence queue overflow", "Datalog type conflict", "Unused", "Unrecognized type (interapplication manager)", "Memory corrupt", "Failed to make temporary DLL", "Old CIN version", "Drag socket not found", "Failed to load drop-object", "Failed to register OLE object", "Failed to release OLE object", "Format specifier type mismatch", "Unknown format specifier", "Too few format specifiers", "Too many format specifiers", "Scan failed", "Newer CIN version", "Error converting to variant", "Runtime menu error", "Password tampered", "Variant attribute not found", "Incompatible variant data type", "Event data is not available", "Event Store is not present", "Occurrence is not found", "Event Queue is not created", "Event info is not available", "Refnum passed is NULL", "Error retrieving Class GUID", "Error retrieving CoClass GUID", "Error retrieving TypeLib GUID.", "Bad built application magic bytes.", "Specific driver is different from the specific driver associated with the Logical Name.", "There is no session opened to the class driver.", "Max Error", "MAX - Error with config objects", "MAX - Error loading configuration", "MAX - Group not supported"]
        # "Current State"
        # "Do not delete, rename, or modify this frame.\n(this is used to capture unhandled states and typos)"
        # "Handle mistyped state name (developer tool)"
        n53 = Format Into String(format string="Software Exception: Unhandled State \"%s\"." ("message"), error in=w152, w147) -> (resulting string=w155:string, error out=w154:errorcluster)  [unwired: 1 in]
        n54 = call <vilib>:"Error Cluster From Error Code.vi"("show call chain? (False)"=TRUE, "error in (no error)"=w154, "error message (\"\")"=w155, "error code (0)"=w156) -> ("error out"=w153:errorcluster)  [unwired: 5 in]
        n55 = call <vilib>:"Add State(s) to Queue__JKI_lib_State_Machine.vi"("State(s) in (\"\")"=w151) -> ("States Out"=w150:string)  [unwired: 14 in]
      }
      frame "Initialize Core Data" {
        # "Do not delete, rename, or modify this frame.\n(this is used to determine panel behavior on exit)"
        # "originally closed?"
        # "exe?"
        # "If panel starts closed or is an EXE, then close it when we exit"
        n56 = property class="VI"() -> ("FP.State"=w162:T5)  [unwired: 2 in, 2 out]
        n57 = control-ref of="Current VI Reference"() -> (w163:refnum<vi>)
        n58 = Equal?(x=w162, y=T5."Closed" ("Front Panel Window:State")) -> (x = y?=w160:bool)
        n59 = property class="App"() -> ("App.Kind"=w168:T6)  [unwired: 2 in, 2 out]
        n60 = Equal?(x=w168, y=T6."Run Time System" ("Application:Kind")) -> (x = y?=w166:bool)
        n61 = Or(x=w160, y=w166) -> (x .or. y?=w164:bool)
        n62 = Bundle By Name(cluster=w165, "Core.Current VI Reference"=w163, "Core.Close Panel on Exit?"=w164) -> (w170:T8)
        n63 = call <vilib>:"Add State(s) to Queue__JKI_lib_State_Machine.vi"("State(s) in (\"\")"=w172) -> ("States Out"=w171:string)  [unwired: 14 in]
      }
      frame "Error Handler" {
        # "Unhandled Error -- Display it"
        # "Handle any errors here.\nYou can also output any states to clean-up after errors occur"
        # "Clear error"
        n64 = call <vilib>:"General Error Handler.vi"("error in (no error)"=w176) -> ()  [unwired: 10 in, 5 out]
        n65 = call <vilib>:"Add State(s) to Queue__JKI_lib_State_Machine.vi"("State(s) in Front (\"\")"="/* Post Error States", "State(s) in (\"\")"=w180) -> ("States Out"=w179:string)  [unwired: 13 in]
      }
      frame "Exit" {
        # "Do not put any code in this frame.\n(No errors that occur here will be handled.)"
        n66 = call <vilib>:"Add State(s) to Queue__JKI_lib_State_Machine.vi"("State(s) in (\"\")"=w187) -> ("States Out"=w186:string)  [unwired: 14 in]
      }
      frame "---------- Data ----------" {
        # "Do not put any code in this frame.\n(It is a separator no-op. You can make a copy of this frame to create a new Data frame)"
        n67 = call <vilib>:"Add State(s) to Queue__JKI_lib_State_Machine.vi"("State(s) in (\"\")"=w193) -> ("States Out"=w192:string)  [unwired: 14 in]
      }
      frame "Data: Initialize" {
        w200 = ""  # 难度_保存
        w196 = 0  # 积分_保存
        w197 = 0  # 闪烁间隔_保存
        w198 = 0  # 超时时间_保存
        w199 = 0  # 亮灯次数_保存
        w201 = ""  # 用户名
        w202 = ""  # 修改密码_账户
        w203 = ""  # 修改密码_新密码
        w204 = ""  # 注册密码
        w205 = T9 {"Current VI Reference"=refnum, "Close Panel on Exit?"=FALSE}  # Core
        w207 = TRUE  # Your Boolean data
        w206 = ""  # 注册账户
        # "do not delete - used by framework"
        # "Add new data here."
        # "Initialize the shift-register data, here.\n(data names are defined by what you wire into the bundle function)"
        n68 = invoke on="选项卡控件" class="TabCtl (严格)" method="Reinit To Default"() -> ()  [unwired: 3 in, 3 out]
        n69 = invoke on="时间到" class="Bool (严格)" method="Reinit To Default"() -> ()  [unwired: 3 in, 3 out]
        n70 = invoke on="上" class="Bool (严格)" method="Reinit To Default"() -> ()  [unwired: 3 in, 3 out]
        n71 = invoke on="左" class="Bool (严格)" method="Reinit To Default"() -> ()  [unwired: 3 in, 3 out]
        n72 = invoke on="右" class="Bool (严格)" method="Reinit To Default"() -> ()  [unwired: 3 in, 3 out]
        n73 = invoke on="下" class="Bool (严格)" method="Reinit To Default"() -> ()  [unwired: 3 in, 3 out]
        n74 = invoke on="亮灯次数" class="DigNum (严格)" method="Reinit To Default"() -> ()  [unwired: 3 in, 3 out]
        n75 = invoke on="分数" class="DigNum (严格)" method="Reinit To Default"() -> ()  [unwired: 3 in, 3 out]
        n76 = invoke on="难度：分数" class="Str" method="Reinit To Default"() -> ()  [unwired: 3 in, 3 out]
        n77 = invoke on="结束" class="Bool (严格)" method="Reinit To Default"() -> ()  [unwired: 3 in, 3 out]
        n78 = invoke on="存档" class="Bool (严格)" method="Reinit To Default"() -> ()  [unwired: 3 in, 3 out]
        n79 = Bundle("Core"=w205, "Your Boolean data"=w207, "注册账户"=w206, "注册密码"=w204, "修改密码_新密码"=w203, "修改密码_账户"=w202, "用户名"=w201, "难度_保存"=w200, "亮灯次数_保存"=w199, "超时时间_保存"=w198, "闪烁间隔_保存"=w197, "积分_保存"=w196) -> (w209:T8)  [unwired: 1 in]
        n80 = call <vilib>:"Add State(s) to Queue__JKI_lib_State_Machine.vi"("State(s) in (\"\")"=w211) -> ("States Out"=w210:string)  [unwired: 14 in]
      }
      frame "Data: Cleanup" {
        # "Cleanup any data and references, here.\n(this is called automatically, by the Macro: Exit)"
        n81 = Unbundle By Name(w214) -> ("Core.Current VI Reference"=w217:refnum<vi>)
        n82 = Close Reference(reference=w217, error in (no error)=w216) -> (error out=w215:errorcluster)
        n83 = call <vilib>:"Add State(s) to Queue__JKI_lib_State_Machine.vi"("State(s) in (\"\")"=w219) -> ("States Out"=w218:string)  [unwired: 14 in]
      }
      frame "---------- UI ----------" {
        # "Do not put any code in this frame.\n(It is a separator no-op. You can make a copy of this frame to create a new UI frame)"
        n84 = call <vilib>:"Add State(s) to Queue__JKI_lib_State_Machine.vi"("State(s) in (\"\")"=w225) -> ("States Out"=w224:string)  [unwired: 14 in]
      }
      frame "UI: Initialize" {
        # "Initialize the User Interface, here.\n(this is called automatically, by the Macro: Init)"
        n85 = invoke on="注册账户" class="Str" method="Reinit To Default"() -> ()  [unwired: 3 in, 3 out]
        n86 = invoke on="账号" class="Str" method="Reinit To Default"() -> ()  [unwired: 3 in, 3 out]
        n87 = invoke on="密码" class="Str" method="Reinit To Default"() -> ()  [unwired: 3 in, 3 out]
        n88 = invoke on="注册密码" class="Str" method="Reinit To Default"() -> ()  [unwired: 3 in, 3 out]
        n89 = invoke on="确认新密码" class="Str" method="Reinit To Default"() -> ()  [unwired: 3 in, 3 out]
        n90 = invoke on="修改密码簇" class="Clust (严格)" method="Reinit To Default"() -> ()  [unwired: 3 in, 3 out]
        n91 = invoke on="用户注册_返回" class="Bool (严格)" method="Reinit To Default"() -> ()  [unwired: 3 in, 3 out]
        n92 = invoke on="用户注册_注册" class="Bool (严格)" method="Reinit To Default"() -> ()  [unwired: 3 in, 3 out]
        n93 = invoke on="修改密码_修改" class="Bool (严格)" method="Reinit To Default"() -> ()  [unwired: 3 in, 3 out]
        n94 = invoke on="修改密码_返回" class="Bool (严格)" method="Reinit To Default"() -> ()  [unwired: 3 in, 3 out]
        n95 = invoke on="主界面_进入游戏" class="Bool (严格)" method="Reinit To Default"() -> ()  [unwired: 3 in, 3 out]
        n96 = invoke on="主界面_返回" class="Bool (严格)" method="Reinit To Default"() -> ()  [unwired: 3 in, 3 out]
        n97 = invoke on="登录界面_登录" class="Bool (严格)" method="Reinit To Default"() -> ()  [unwired: 3 in, 3 out]
        n98 = invoke on="登录界面_退出" class="Bool (严格)" method="Reinit To Default"() -> ()  [unwired: 3 in, 3 out]
        n99 = invoke on="登陆界面_注册" class="Bool (严格)" method="Reinit To Default"() -> ()  [unwired: 3 in, 3 out]
        n100 = invoke on="登录界面_修改密码" class="Bool (严格)" method="Reinit To Default"() -> ()  [unwired: 3 in, 3 out]
        n101 = invoke on="游戏规则_返回" class="Bool (严格)" method="Reinit To Default"() -> ()  [unwired: 3 in, 3 out]
        n102 = invoke on="TOP10_返回" class="Bool (严格)" method="Reinit To Default"() -> ()  [unwired: 3 in, 3 out]
        n103 = call <vilib>:"Add State(s) to Queue__JKI_lib_State_Machine.vi"("State(s) in (\"\")"=w231) -> ("States Out"=w230:string)  [unwired: 14 in]
      }
      frame "UI: Cursor Set" {
        # "Argument"
        # "Set and Unset Cursor Busy.\n(Usage: \"UI: Cursor Set >> Busy|Idle\")"
        n104 = case shown="\"Idle\", 默认" w234 {
          tunnel: w236 -> [w241 w243]
          tunnel: [w240 w242] -> w235
          frame "Idle", Default {
            n105 = call <vilib>:"Unset Busy.vi"("error in (no error)"=w241) -> ("error out"=w240:errorcluster)  [unwired: 10 in]
          }
          frame "Busy" {
            n106 = call <vilib>:"Set Busy.vi"("error in (no error)"=w243) -> ("error out"=w242:errorcluster)  [unwired: 9 in, 1 out]
          }
        }
        n107 = call <vilib>:"Add State(s) to Queue__JKI_lib_State_Machine.vi"("State(s) in (\"\")"=w239) -> ("States Out"=w238:string)  [unwired: 14 in]
      }
      frame "UI: Front Panel State" {
        # "Argument"
        # "Set Front Panel Open or Closed\n(Usage: \"UI: Front Panel State >> Open|Close\")"
        n108 = Unbundle By Name(w248) -> ("Core.Current VI Reference"=w247:refnum<vi>)
        n109 = case shown="\"Open\", \"Standard\", 默认" w246 {
          tunnel: w250 -> [w258 w273 w284 w297 w310]
          tunnel: [w260 w274 w286 w299 w312] -> w249
          tunnel: w247 -> [w259 w271 w285 w298 w311]
          frame "Open", "Standard", Default {
            w253 = T5."Standard" ("State")
            n110 = property class="VI"(reference=w259, error in=w258) -> (reference out=w256:refnum<vi>, error out=w257:errorcluster, "FP.State"=w255:T5)
            n111 = Not Equal?(x=w255, y=w253) -> (x != y?=w254:bool)
            n112 = case shown="假" w254 {
              tunnel: [w264 w266] -> w260
              tunnel: w257 -> [w263 w266]
              tunnel: w256 -> [w262 _]
              tunnel: w253 -> [w261 _]
              frame True {
                n113 = invoke class="VI" method="FP.Open"(reference=w262, error in=w263, "Activate"=TRUE, "State"=w261) -> (error out=w264:errorcluster)  [unwired: 1 in, 4 out]
              }
              frame False {
              }
            }
          }
          frame "Close", "Closed" {
            n114 = property class="VI"(reference=w271, error in=w273) -> (reference out=w270:refnum<vi>, error out=w272:errorcluster, "FP.State"=w268:T5)
            n115 = Not Equal?(x=w268, y=T5."Closed" ("Front Panel Window:State")) -> (x != y?=w267:bool)
            n116 = case shown="真" w267 {
              tunnel: [w275 w278] -> w274
              tunnel: w272 -> [w275 w277]
              tunnel: w270 -> [_ w276]
              frame False {
              }
              frame True {
                n117 = invoke class="VI" method="FP.Close"(reference=w276, error in=w277) -> (error out=w278:errorcluster)  [unwired: 1 in, 2 out]
              }
            }
          }
          frame "Hidden", "Hide" {
            w279 = T5."Hidden" ("State")
            n118 = property class="VI"(reference=w285, error in=w284) -> (reference out=w282:refnum<vi>, error out=w283:errorcluster, "FP.State"=w281:T5)
            n119 = Not Equal?(x=w281, y=w279) -> (x != y?=w280:bool)
            n120 = case shown="真" w280 {
              tunnel: [w290 w291] -> w286
              tunnel: w283 -> [w289 w291]
              tunnel: w282 -> [w288 _]
              tunnel: w279 -> [w287 _]
              frame True {
                n121 = invoke class="VI" method="FP.Open"(reference=w288, error in=w289, "State"=w287) -> (error out=w290:errorcluster)  [unwired: 2 in, 4 out]
              }
              frame False {
              }
            }
          }
          frame "Minimize", "Minimized" {
            w292 = T5."Minimized" ("State")
            n122 = property class="VI"(reference=w298, error in=w297) -> (reference out=w295:refnum<vi>, error out=w296:errorcluster, "FP.State"=w294:T5)
            n123 = Not Equal?(x=w294, y=w292) -> (x != y?=w293:bool)
            n124 = case shown="真" w293 {
              tunnel: [w303 w304] -> w299
              tunnel: w296 -> [w302 w304]
              tunnel: w295 -> [w301 _]
              tunnel: w292 -> [w300 _]
              frame True {
                n125 = invoke class="VI" method="FP.Open"(reference=w301, error in=w302, "State"=w300) -> (error out=w303:errorcluster)  [unwired: 2 in, 4 out]
              }
              frame False {
              }
            }
          }
          frame "Maximize", "Maximized" {
            w305 = T5."Maximized" ("State")
            n126 = property class="VI"(reference=w311, error in=w310) -> (reference out=w308:refnum<vi>, error out=w309:errorcluster, "FP.State"=w307:T5)
            n127 = Not Equal?(x=w307, y=w305) -> (x != y?=w306:bool)
            n128 = case shown="真" w306 {
              tunnel: [w316 w317] -> w312
              tunnel: w309 -> [w315 w317]
              tunnel: w308 -> [w314 _]
              tunnel: w305 -> [w313 _]
              frame True {
                n129 = invoke class="VI" method="FP.Open"(reference=w314, error in=w315, "State"=w313) -> (error out=w316:errorcluster)  [unwired: 2 in, 4 out]
              }
              frame False {
              }
            }
          }
        }
        n130 = call <vilib>:"Add State(s) to Queue__JKI_lib_State_Machine.vi"("State(s) in (\"\")"=w252) -> ("States Out"=w251:string)  [unwired: 14 in]
      }
      frame "---------- Macro ----------" {
        # "Do not put any code in this frame.\n(It is a separator no-op. You can make a copy of this frame to create a new Macro frame)"
        n131 = call <vilib>:"Add State(s) to Queue__JKI_lib_State_Machine.vi"("State(s) in (\"\")"=w323) -> ("States Out"=w322:string)  [unwired: 14 in]
      }
      frame "Macro: Initialize" {
        # "Initialization Macro\n(This is called once, when the VI starts)"
        n132 = call <vilib>:"Add State(s) to Queue__JKI_lib_State_Machine.vi"("State(s) in Front (\"\")"="Data: Initialize\nInitialize Core Data\nUI: Initialize\nUI: Front Panel State >> Open", "State(s) in (\"\")"=w330) -> ("States Out"=w329:string)  [unwired: 13 in]
      }
      frame "Macro: Exit" {
        # "Exit Macro\n(This is called once, when the VI exits)"
        n133 = Unbundle By Name(w339) -> ("Core.Close Panel on Exit?"=w338:bool)
        n134 = Select(t="UI: Front Panel State >> Close", s=w338, f="") -> (s? t:f=w335:string)
        n135 = call <vilib>:"Add State(s) to Queue__JKI_lib_State_Machine.vi"("State(s) in (\"\")"=w335, "State(s) at Back (\"\")"="Data: Cleanup\nExit") -> ("States Out"=w333:string)  [unwired: 13 in]
        n136 = call <vilib>:"Add State(s) to Queue__JKI_lib_State_Machine.vi"("State(s) in Front (\"\")"=w333, "State(s) in (\"\")"=w342) -> ("States Out"=w341:string)  [unwired: 13 in]
      }
      frame "---------- User ----------" {
        # "Template Separator\n(You can make a copy of, or modify, this frame)"
        n137 = call <vilib>:"Add State(s) to Queue__JKI_lib_State_Machine.vi"("State(s) in (\"\")"=w348) -> ("States Out"=w347:string)  [unwired: 14 in]
      }
      frame "User: modify_password" {
        # "Template Separator\n(You can make a copy of, or modify, this frame)"
        n138 = event shown="[0] \"修改密码_修改\": 鼠标按下" {
          selector: _ -> [_ _ _]
          dyn-events: _ -> [_ _ _]
          timeout: 100 -> [_ _ _]
          tunnel: [w378 "User: modify_password" "Idle"] -> w354
          tunnel: w353 -> [w365 w435 w437]
          tunnel: [w364 w435 w437] -> w352
          event "修改密码_修改": Mouse Down {
            n139 = event-data() -> ()  [unwired: 1 in, 8 out]
            n140 = call <vilib>:"Application Directory.vi"() -> ("Application Directory"=w382:path)
            n141 = Build Path(base path=w382, name or relative path="账户信息.txt" ("名称或相对路径")) -> (appended path=w381:path)
            n142 = call-poly <vilib>:"Read Delimited Spreadsheet.vi"("file path (dialog if empty)"=w381) -> ("all rows"=w375:string[][])  [unwired: 9 in, 5 out]
            n143 = Unbundle By Name("修改密码簇") -> ("账号"=w361:string, "旧密码"=w371:string, "新密码"=w359:string, "确认密码"=w363:string)  [unwired: 1 out]
            n144 = Wait (ms)(milliseconds to wait=u32 50 ("等待时间（毫秒）")) -> ()  [unwired: 1 out]
            n145 = Index Array(array=w375, index (col)=0 ("禁用的索引 (列)")) -> (element=w377:string[])  [unwired: 1 in]
            n146 = Equal?(x=w371, y=w359) -> (x = y?=w379:bool)
            n147 = Equal?(x=w359, y=w363) -> (x = y?=w362:bool)
            n148 = Search 1D Array(1D array=w377, element=w361) -> (index of element=w374:i32)  [unwired: 1 in]
            n149 = String Length(string=w359) -> (length=w370:i32)
            n150 = Equal?(x=w370, y=0) -> (x = y?=w368:bool)
            n151 = Index Array(array=w375, index (row)=w374, index (col)=1 ("禁用的索引 (列)")) -> (element=w372:string)
            n152 = Equal?(x=w372, y=w371) -> (x = y?=w366:bool)
            n153 = Equal?(x=w374, y=-1) -> (x = y?=w367:bool)
            n154 = case shown="假" w379 {
              tunnel: [w391 "User: modify_password" ("消息")] -> w378
              tunnel: w368 -> [w392 _]
              tunnel: w367 -> [w390 _]
              tunnel: w366 -> [w389 _]
              tunnel: w365 -> [w388 w431]
              tunnel: w359 -> [w387 _]
              tunnel: [w386 w431] -> w364
              tunnel: w362 -> [w385 _]
              tunnel: w361 -> [w384 _]
              frame False {
                n155 = case shown="假" w392 {
                  tunnel: [w399 "User: modify_password" ("消息")] -> w391
                  tunnel: w390 -> [w400 _]
                  tunnel: w389 -> [w398 _]
                  tunnel: w388 -> [w397 w428]
                  tunnel: w387 -> [w396 _]
                  tunnel: [w395 w428] -> w386
                  tunnel: w385 -> [w394 _]
                  tunnel: w384 -> [w393 _]
                  frame False {
                    n156 = case shown="假" w400 {
                      tunnel: [w406 "User: modify_password" ("消息")] -> w399
                      tunnel: w398 -> [w407 _]
                      tunnel: w397 -> [w405 w425]
                      tunnel: w396 -> [w404 _]
                      tunnel: [w403 w425] -> w395
                      tunnel: w394 -> [w402 _]
                      tunnel: w393 -> [w401 _]
                      frame False {
                        n157 = case shown="真" w407 {
                          tunnel: ["User: modify_password" ("消息") w415] -> w406
                          tunnel: w405 -> [w408 w414]
                          tunnel: w404 -> [_ w413]
                          tunnel: [w408 w412] -> w403
                          tunnel: w402 -> [_ w416]
                          tunnel: w401 -> [_ w411]
                          frame False {
                            n158 = One Button Dialog(message="账户或密码错误" ("消息")) -> ()  [unwired: 1 in, 1 out]
                          }
                          frame True {
                            n159 = case shown="真" w416 {
                              tunnel: ["User: modify_password" ("消息") "User: Info >> modify" ("消息")] -> w415
                              tunnel: w414 -> [w417 w423]
                              tunnel: w413 -> [_ w422]
                              tunnel: [w417 w421] -> w412
                              tunnel: w411 -> [_ w420]
                              frame False {
                                n160 = One Button Dialog(message="两次密码不一致" ("消息")) -> ()  [unwired: 1 in, 1 out]
                              }
                              frame True {
                                n161 = Bundle By Name(cluster=w423, "修改密码_账户"=w420, "修改密码_新密码"=w422) -> (w421:T8)
                              }
                            }
                          }
                        }
                      }
                      frame True {
                        n162 = One Button Dialog(message="用户不存在" ("消息")) -> ()  [unwired: 1 in, 1 out]
                      }
                    }
                  }
                  frame True {
                    n163 = One Button Dialog(message="新密码不能为空" ("消息")) -> ()  [unwired: 1 in, 1 out]
                  }
                }
              }
              frame True {
                n164 = One Button Dialog(message="新密码与旧密码不能相同" ("消息")) -> ()  [unwired: 1 in, 1 out]
              }
            }
          }
          event Timeout {
            n165 = event-data() -> ()  [unwired: 1 in, 3 out]
          }
          event "修改密码_返回": Value Change {
            n166 = event-data() -> ()  [unwired: 1 in, 6 out]
            n167 = local write "选项卡控件"(选项卡枚举."登录界面" ("枚举")) -> ()
          }
        }
        n168 = call <vilib>:"Add State(s) to Queue__JKI_lib_State_Machine.vi"("State(s) in (\"\")"=w357, "State(s) at Back (\"\")"=w354) -> ("States Out"=w356:string)  [unwired: 13 in]
      }
      frame "User: Info" {
        # "Template Separator\n(You can make a copy of, or modify, this frame)"
        n169 = case shown="\"register\"" w441 {
          tunnel: w444 -> [w461 w470]
          tunnel: ["UI: Initialize" "UI: Initialize"] -> w443
          frame "modify", Default {
            n170 = Unbundle By Name(w461) -> ("修改密码_账户"=w451:string, "修改密码_新密码"=w456:string)
            n171 = call <vilib>:"Application Directory.vi"() -> ("Application Directory"=w463:path)
            n172 = local write "选项卡控件"(选项卡枚举."登录界面" ("枚举")) -> ()
            n173 = Build Array(w451, w456) -> (w455:string[])
            n174 = Build Path(base path=w463, name or relative path="账户信息.txt" ("名称或相对路径")) -> (appended path=w454:path)
            n175 = Concatenate Strings("用户“" ("字符串"), w451, "”密码修改成功" ("字符串")) -> (w449:string)
            n176 = One Button Dialog(message=w449) -> ()  [unwired: 1 in, 1 out]
            n177 = call-poly <vilib>:"Read Delimited Spreadsheet.vi"("file path (dialog if empty)"=w454) -> ("all rows"=w458:string[][])  [unwired: 9 in, 5 out]
            n178 = Index Array(array=w458, index (col)=0 ("禁用的索引 (列)")) -> (element=w459:string[])  [unwired: 1 in]
            n179 = Search 1D Array(1D array=w459, element=w451) -> (index of element=w457:i32)  [unwired: 1 in]
            n180 = Replace Array Subset(array=w458, new element=w455, index (row)=w457) -> (w453:string[][])  [unwired: 1 in]
            n181 = call-poly <vilib>:"Write Delimited Spreadsheet.vi"("file path (dialog if empty)"=w454, "2D data"=w453) -> ()  [unwired: 12 in, 2 out]
          }
          frame "register" {
            n182 = Unbundle By Name(w470) -> ("注册账户"=w469:string, "注册密码"=w468:string)
            n183 = Build Array(w469, w468) -> (w467:string[])
            n184 = call <vilib>:"Application Directory.vi"() -> ("Application Directory"=w474:path)
            n185 = local write "选项卡控件"(选项卡枚举."登录界面" ("枚举")) -> ()
            n186 = Build Path(base path=w474, name or relative path="账户信息.txt" ("名称或相对路径")) -> (appended path=w472:path)
            n187 = call-poly <vilib>:"Write Delimited Spreadsheet.vi"("file path (dialog if empty)"=w472, "1D data"=w467, "append to file? (new file:F)"=TRUE) -> ()  [unwired: 11 in, 2 out]
          }
        }
        n188 = Wait (ms)(milliseconds to wait=u32 50 ("等待时间（毫秒）")) -> ()  [unwired: 1 out]
        n189 = call <vilib>:"Add State(s) to Queue__JKI_lib_State_Machine.vi"("State(s) in (\"\")"=w447, "State(s) at Back (\"\")"=w443) -> ("States Out"=w446:string)  [unwired: 13 in]
      }
      frame "User: register" {
        # "Template Separator\n(You can make a copy of, or modify, this frame)"
        n190 = event shown="[0] \"用户注册_注册\": 鼠标按下" {
          selector: _ -> [_ _ _]
          dyn-events: _ -> [_ _ _]
          timeout: 100 -> [_ _ _]
          tunnel: [w506 "User: register" "Idle"] -> w480
          tunnel: w479 -> [w489 w537 w540]
          tunnel: [w486 w537 w540] -> w478
          event "用户注册_注册": Mouse Down {
            w493 = 0 ("y")
            n191 = event-data() -> ()  [unwired: 1 in, 1 out]
            n192 = call <vilib>:"Application Directory.vi"() -> ("Application Directory"=w501:path)
            n193 = Build Path(base path=w501, name or relative path="账户信息.txt" ("名称或相对路径")) -> (appended path=w502:path)
            n194 = Unbundle By Name("注册簇") -> ("注册账户"=w488:string, "注册密码"=w487:string, "确认密码"=w498:string)
            n195 = call-poly <vilib>:"Read Delimited Spreadsheet.vi"("file path (dialog if empty)"=w502) -> ("all rows"=w503:string[][])  [unwired: 9 in, 5 out]
            n196 = Equal?(x=w487, y=w498) -> (x = y?=w507:bool)
            n197 = String Length(string=w488) -> (length=w494:i32)
            n198 = String Length(string=w487) -> (length=w505:i32)
            n199 = Index Array(array=w503, index (col)=0 ("禁用的索引 (列)")) -> (element=w504:string[])  [unwired: 1 in]
            n200 = Equal?(x=w494, y=w493) -> (x = y?=w491:bool)
            n201 = Equal?(x=w505, y=w493) -> (x = y?=w492:bool)
            n202 = Search 1D Array(1D array=w504, element=w488) -> (index of element=w497:i32)  [unwired: 1 in]
            n203 = Or(x=w491, y=w492) -> (x .or. y?=w490:bool)
            n204 = Equal?(x=w497, y=-1) -> (x = y?=w495:bool)
            n205 = case shown="真" w507 {
              tunnel: ["User: register" w516] -> w506
              tunnel: w490 -> [_ w517]
              tunnel: w495 -> [_ w515]
              tunnel: w489 -> [w508 w514]
              tunnel: w488 -> [_ w513]
              tunnel: w487 -> [_ w512]
              tunnel: [w508 w511] -> w486
              frame False {
                n206 = One Button Dialog(message="两次密码不一致" ("消息")) -> ()  [unwired: 1 in, 1 out]
              }
              frame True {
                n207 = case shown="假" w517 {
                  tunnel: [w522 "User: register"] -> w516
                  tunnel: w515 -> [w523 _]
                  tunnel: w514 -> [w521 w534]
                  tunnel: w513 -> [w520 _]
                  tunnel: w512 -> [w519 _]
                  tunnel: [w518 w534] -> w511
                  frame False {
                    n208 = case shown="真" w523 {
                      tunnel: ["User: register" "User: Info >> register"] -> w522
                      tunnel: w521 -> [w524 w531]
                      tunnel: w520 -> [_ w530]
                      tunnel: w519 -> [_ w529]
                      tunnel: [w524 w528] -> w518
                      frame False {
                        n209 = One Button Dialog(message="账户已存在" ("消息")) -> ()  [unwired: 1 in, 1 out]
                      }
                      frame True {
                        n210 = Bundle By Name(cluster=w531, "注册账户"=w530, "注册密码"=w529) -> (w528:T8)
                        n211 = local write "选项卡控件"(选项卡枚举."登录界面" ("枚举")) -> ()
                        n212 = One Button Dialog(message="注册成功！" ("消息")) -> ()  [unwired: 1 in, 1 out]
                      }
                    }
                  }
                  frame True {
                    n213 = One Button Dialog(message="账户或密码不能为空！" ("消息")) -> ()  [unwired: 1 in, 1 out]
                  }
                }
              }
            }
            n214 = Wait (ms)(milliseconds to wait=u32 50 ("等待时间（毫秒）")) -> ()  [unwired: 1 out]
          }
          event Timeout {
            n215 = event-data() -> ()  [unwired: 1 in, 3 out]
          }
          event "用户注册_返回": Mouse Down {
            n216 = event-data() -> ()  [unwired: 1 in, 8 out]
            n217 = local write "选项卡控件"(选项卡枚举."登录界面" ("枚举")) -> ()
          }
        }
        n218 = call <vilib>:"Add State(s) to Queue__JKI_lib_State_Machine.vi"("State(s) in (\"\")"=w483, "State(s) at Back (\"\")"=w480) -> ("States Out"=w482:string)  [unwired: 13 in]
      }
      frame "User: login" {
        w554 = 0 ("y")
        # "根据账户索引获取密码"
        # "查询账户，获取账户索引"
        # "Your code here.\n(You can make a copy of, or modify, this frame)"
        n219 = call <vilib>:"Application Directory.vi"() -> ("Application Directory"=w566:path)
        n220 = Build Path(base path=w566, name or relative path="账户信息.txt" ("名称或相对路径")) -> (appended path=w564:path)
        n221 = call-poly <vilib>:"Read Delimited Spreadsheet.vi"("file path (dialog if empty)"=w564) -> ("all rows"=w558:string[][])  [unwired: 9 in, 5 out]
        n222 = Index Array(array=w558, index (col)=0 ("禁用的索引 (列)")) -> (element=w562:string[])  [unwired: 1 in]
        n223 = Search 1D Array(1D array=w562, element="账号") -> (index of element=w560:i32)  [unwired: 1 in]
        n224 = String Length(string="账号") -> (length=w556:i32)
        n225 = String Length(string="密码") -> (length=w555:i32)
        n226 = Equal?(x=w556, y=w554) -> (x = y?=w553:bool)
        n227 = Equal?(x=w555, y=w554) -> (x = y?=w552:bool)
        n228 = Equal?(x=w560, y=-1) -> (x = y?=w549:bool)
        n229 = Index Array(array=w558, index (row)=w560, index (col)=1 ("索引 (列)")) -> (element=w557:string)
        n230 = Equal?(x=w557, y="密码") -> (x = y?=w548:bool)
        n231 = Or(x=w553, y=w552) -> (x .or. y?=w551:bool)
        n232 = case shown="假" w551 {
          tunnel: [w574 "Idle" ("State(s) at Back (\"\")")] -> w550
          tunnel: w549 -> [w575 _]
          tunnel: w548 -> [w573 _]
          tunnel: w547 -> [w572 w593]
          tunnel: [w571 w593] -> w546
          tunnel: "账号" -> [w570 _]
          frame False {
            n233 = case shown="假" w575 {
              tunnel: [w579 "Idle"] -> w574
              tunnel: w573 -> [w580 _]
              tunnel: w572 -> [w578 w590]
              tunnel: [w577 w590] -> w571
              tunnel: w570 -> [w576 _]
              frame False {
                n234 = case shown="真" w580 {
                  tunnel: ["Idle" "Idle"] -> w579
                  tunnel: w578 -> [w581 w586]
                  tunnel: [w581 w585] -> w577
                  tunnel: w576 -> [_ w584]
                  frame False {
                    n235 = One Button Dialog(message="用户名或密码错误" ("消息")) -> ()  [unwired: 1 in, 1 out]
                  }
                  frame True {
                    n236 = Bundle By Name(cluster=w586, "用户名"=w584) -> (w585:T8)
                    n237 = One Button Dialog(message="登录成功" ("消息")) -> ()  [unwired: 1 in, 1 out]
                    n238 = local write "选项卡控件"(选项卡枚举."主界面" ("枚举")) -> ()
                  }
                }
              }
              frame True {
                n239 = One Button Dialog(message="用户名不存在" ("消息")) -> ()  [unwired: 1 in, 1 out]
              }
            }
          }
          frame True {
            n240 = One Button Dialog(message="用户名或密码不能为空！" ("消息")) -> ()  [unwired: 1 in, 1 out]
          }
        }
        n241 = call <vilib>:"Add State(s) to Queue__JKI_lib_State_Machine.vi"("State(s) in (\"\")"=w569, "State(s) at Back (\"\")"=w550) -> ("States Out"=w568:string)  [unwired: 13 in]
      }
      frame "User: Exit" {
        # "Your code here.\n(You can make a copy of, or modify, this frame)"
        n242 = call <vilib>:"Add State(s) to Queue__JKI_lib_State_Machine.vi"("State(s) in (\"\")"=w601) -> ("States Out"=w600:string)  [unwired: 14 in]
      }
      frame "---------- Game ----------" {
        # "Template Separator\n(You can make a copy of, or modify, this frame)"
        n243 = call <vilib>:"Add State(s) to Queue__JKI_lib_State_Machine.vi"("State(s) in (\"\")"=w607) -> ("States Out"=w606:string)  [unwired: 14 in]
      }
      frame "Game: Select_Difficulty" {
        # "Template Separator\n(You can make a copy of, or modify, this frame)"
        n244 = Concatenate Strings("欢迎" ("message"), "选择难度" ("string"), "\r") -> (w618:string)
        n245 = call <vilib>:"Three Button Dialog.vi"("Allow user to close window? (TRUE)"=FALSE, "Right Button Text (\"Cancel\")"="困难" ("Right Button Text (\"Cancel\")"), "Center Button Text (\"No\")"="中等" ("Center Button Text (\"No\")"), "Left Button Text (\"Yes\")"="简单" ("Left Button Text (\"Yes\")"), "message"=w618) -> ("Which Button?"=w616:T10)  [unwired: 6 in]
        n246 = case shown="\"Center Button\"" w616 {
          tunnel: [727 484 303] -> w611
          tunnel: [750 550 350] -> w612
          tunnel: ["简单" "中等" "困难"] -> w613
          frame "Left Button", Default {
          }
          frame "Center Button" {
          }
          frame "Right Button" {
          }
        }
        "超时时间" <- w611
        "闪烁间隔" <- w612
        "难度" <- w613
        n247 = Bundle By Name(cluster=w615, "难度_保存"=w613, "闪烁间隔_保存"=w612, "超时时间_保存"=w611) -> (w614:T8)
        n248 = call <vilib>:"Add State(s) to Queue__JKI_lib_State_Machine.vi"("State(s) in (\"\")"=w627, "State(s) at Back (\"\")"="Game: Twinkle" ("State(s) at Back (\"\")")) -> ("States Out"=w626:string)  [unwired: 13 in]
      }
      frame "Game: Twinkle" {
        # "根据回合选择亮灯顺序"
        # "Template Separator\n(You can make a copy of, or modify, this frame)"
        n249 = Array Subset(array=w641, index=0 ("索引"), length="亮灯次数") -> (w639:u64[])
        n250 = for {
          tunnel: w639 -> [w647] mode=indexing
          stop <- w648 stop-if-true
          n251 = case shown="1" w647 {
            frame 0, Default {
              n252 = stacked-sequence {
                frame #0 {
                  n253 = local write "上"(TRUE ("上")) -> ()
                }
                frame #1 {
                  n254 = local read "闪烁间隔"() -> (w650:i32)
                  n255 = Wait (ms)(milliseconds to wait=w650) -> ()  [unwired: 1 out]
                }
                frame #2 {
                  n256 = local write "上"(FALSE ("上")) -> ()
                }
                frame #3 {
                  n257 = Wait (ms)(milliseconds to wait=u32 250 ("等待时间（毫秒）")) -> ()  [unwired: 1 out]
                }
              }
            }
            frame 1 {
              n258 = stacked-sequence {
                frame #0 {
                  n259 = local write "右"(TRUE ("上")) -> ()
                }
                frame #1 {
                  n260 = local read "闪烁间隔"() -> (w654:i32)
                  n261 = Wait (ms)(milliseconds to wait=w654) -> ()  [unwired: 1 out]
                }
                frame #2 {
                  n262 = local write "右"(FALSE ("上")) -> ()
                }
                frame #3 {
                  n263 = Wait (ms)(milliseconds to wait=u32 250 ("等待时间（毫秒）")) -> ()  [unwired: 1 out]
                }
              }
            }
            frame 2 {
              n264 = stacked-sequence {
                frame #0 {
                  n265 = local write "下"(TRUE ("上")) -> ()
                }
                frame #1 {
                  n266 = local read "闪烁间隔"() -> (w658:i32)
                  n267 = Wait (ms)(milliseconds to wait=w658) -> ()  [unwired: 1 out]
                }
                frame #2 {
                  n268 = local write "下"(FALSE ("上")) -> ()
                }
                frame #3 {
                  n269 = Wait (ms)(milliseconds to wait=u32 250 ("等待时间（毫秒）")) -> ()  [unwired: 1 out]
                }
              }
            }
            frame 3 {
              n270 = stacked-sequence {
                frame #0 {
                  n271 = local write "左"(TRUE ("上")) -> ()
                }
                frame #1 {
                  n272 = local read "闪烁间隔"() -> (w662:i32)
                  n273 = Wait (ms)(milliseconds to wait=w662) -> ()  [unwired: 1 out]
                }
                frame #2 {
                  n274 = local write "左"(FALSE ("上")) -> ()
                }
                frame #3 {
                  n275 = Wait (ms)(milliseconds to wait=u32 250 ("等待时间（毫秒）")) -> ()  [unwired: 1 out]
                }
              }
            }
          }
          n276 = local read "结束"() -> (w648:bool)
        }
        n277 = call <vilib>:"Add State(s) to Queue__JKI_lib_State_Machine.vi"("State(s) in (\"\")"=w646, "State(s) at Back (\"\")"="Game: start counting" ("State(s) at Back (\"\")")) -> ("States Out"=w645:string)  [unwired: 13 in]
      }
      frame "Game: start counting" {
        # "Template Separator\n(You can make a copy of, or modify, this frame)"
        n278 = local write "是否开始计时？"(TRUE ("是否开始计时？")) -> ()
        n279 = call <vilib>:"Add State(s) to Queue__JKI_lib_State_Machine.vi"("State(s) in (\"\")"=w672, "State(s) at Back (\"\")"="Game: Option" ("State(s) at Back (\"\")")) -> ("States Out"=w671:string)  [unwired: 13 in]
      }
      frame "Game: Option" {
        # "提取要判断的灯号"
        # "判断是否超时"
        # "判断点亮的灯是否正确\n+1使判断的索引每循环一次向后移一位"
        # "判断是否按完"
        # "Template Separator\n(You can make a copy of, or modify, this frame)"
        n280 = Decrement(x=w685) -> (x-1=w686:i32)
        n281 = Index Array(array=w684, index=w686) -> (element=w681:u64)
        n282 = event shown="[6] \"右\": 鼠标按下" {
          selector: _ -> [_ _ _ _ _ _ _ _ _ _]
          dyn-events: _ -> [_ _ _ _ _ _ _ _ _ _]
          timeout: 10000 -> [_ _ _ _ _ _ _ _ _ _]
          tunnel: [按键枚举."绿" 按键枚举."退出" w754 按键枚举."红" 按键枚举."存档" 按键枚举."读档" 按键枚举."蓝" 按键枚举."黄" 按键枚举."按错" 按键枚举."退出"] -> w680
          tunnel: w685 -> [w746 w752 w753 w778 w784 w786 w788 w794 w800 w803]
          tunnel: [w746 w752 w753 w778 w784 w786 w788 w794 w800 w803] -> w682
          event "上": Mouse Down {
            n283 = event-data() -> ()  [unwired: 1 in, 1 out]
            n284 = stacked-sequence {
              frame #0 {
                n285 = local write "上"(TRUE ("上")) -> ()
              }
              frame #1 {
                n286 = Wait (ms)(milliseconds to wait=u32 60 ("等待时间（毫秒）")) -> ()  [unwired: 1 out]
              }
              frame #2 {
                n287 = local write "上"(FALSE ("上")) -> ()
              }
              frame #3 {
                n288 = Wait (ms)(milliseconds to wait=u32 60 ("等待时间（毫秒）")) -> ()  [unwired: 1 out]
              }
            }
          }
          event "结束": Value Change {
            n289 = event-data() -> ()  [unwired: 1 in, 1 out]
          }
          event Key Down {
            n290 = event-data() -> ("VKey"=w755:T11)  [unwired: 1 in]
            n291 = case shown="\"ASCII\", 默认" w755 {
              tunnel: [按键枚举."按错" 按键枚举."绿" 按键枚举."蓝" 按键枚举."红" 按键枚举."黄"] -> w754
              frame "ASCII", Default {
              }
              frame "Up" {
                n292 = stacked-sequence {
                  frame #0 {
                    n293 = local write "上"(TRUE ("上")) -> ()
                  }
                  frame #1 {
                    n294 = Wait (ms)(milliseconds to wait=u32 60 ("等待时间（毫秒）")) -> ()  [unwired: 1 out]
                  }
                  frame #2 {
                    n295 = local write "上"(FALSE ("上")) -> ()
                  }
                  frame #3 {
                    n296 = Wait (ms)(milliseconds to wait=u32 60 ("等待时间（毫秒）")) -> ()  [unwired: 1 out]
                  }
                }
              }
              frame "Right" {
                n297 = stacked-sequence {
                  frame #0 {
                    n298 = local write "右"(TRUE ("上")) -> ()
                  }
                  frame #1 {
                    n299 = Wait (ms)(milliseconds to wait=u32 60 ("等待时间（毫秒）")) -> ()  [unwired: 1 out]
                  }
                  frame #2 {
                    n300 = local write "右"(FALSE ("上")) -> ()
                  }
                  frame #3 {
                    n301 = Wait (ms)(milliseconds to wait=u32 60 ("等待时间（毫秒）")) -> ()  [unwired: 1 out]
                  }
                }
              }
              frame "Down" {
                n302 = stacked-sequence {
                  frame #0 {
                    n303 = local write "下"(TRUE ("上")) -> ()
                  }
                  frame #1 {
                    n304 = Wait (ms)(milliseconds to wait=u32 60 ("等待时间（毫秒）")) -> ()  [unwired: 1 out]
                  }
                  frame #2 {
                    n305 = local write "下"(FALSE ("上")) -> ()
                  }
                  frame #3 {
                    n306 = Wait (ms)(milliseconds to wait=u32 60 ("等待时间（毫秒）")) -> ()  [unwired: 1 out]
                  }
                }
              }
              frame "Left" {
                n307 = stacked-sequence {
                  frame #0 {
                    n308 = local write "左"(TRUE ("上")) -> ()
                  }
                  frame #1 {
                    n309 = Wait (ms)(milliseconds to wait=u32 60 ("等待时间（毫秒）")) -> ()  [unwired: 1 out]
                  }
                  frame #2 {
                    n310 = local write "左"(FALSE ("上")) -> ()
                  }
                  frame #3 {
                    n311 = Wait (ms)(milliseconds to wait=u32 60 ("等待时间（毫秒）")) -> ()  [unwired: 1 out]
                  }
                }
              }
            }
          }
          event "下": Mouse Down {
            n312 = event-data() -> ()  [unwired: 1 in, 1 out]
            n313 = stacked-sequence {
              frame #0 {
                n314 = local write "下"(TRUE ("上")) -> ()
              }
              frame #1 {
                n315 = Wait (ms)(milliseconds to wait=u32 60 ("等待时间（毫秒）")) -> ()  [unwired: 1 out]
              }
              frame #2 {
                n316 = local write "下"(FALSE ("上")) -> ()
              }
              frame #3 {
                n317 = Wait (ms)(milliseconds to wait=u32 60 ("等待时间（毫秒）")) -> ()  [unwired: 1 out]
              }
            }
          }
          event "存档": Mouse Down {
            n318 = event-data() -> ()  [unwired: 1 in, 1 out]
          }
          event "读档": Mouse Down {
            n319 = event-data() -> ()  [unwired: 1 in, 1 out]
          }
          event "右": Mouse Down {
            n320 = event-data() -> ()  [unwired: 1 in, 1 out]
            n321 = stacked-sequence {
              frame #0 {
                n322 = local write "右"(TRUE ("上")) -> ()
              }
              frame #1 {
                n323 = Wait (ms)(milliseconds to wait=u32 60 ("等待时间（毫秒）")) -> ()  [unwired: 1 out]
              }
              frame #2 {
                n324 = local write "右"(FALSE ("上")) -> ()
              }
              frame #3 {
                n325 = Wait (ms)(milliseconds to wait=u32 60 ("等待时间（毫秒）")) -> ()  [unwired: 1 out]
              }
            }
          }
          event "左": Mouse Down {
            n326 = event-data() -> ()  [unwired: 1 in, 1 out]
            n327 = stacked-sequence {
              frame #0 {
                n328 = local write "左"(TRUE ("上")) -> ()
              }
              frame #1 {
                n329 = Wait (ms)(milliseconds to wait=u32 60 ("等待时间（毫秒）")) -> ()  [unwired: 1 out]
              }
              frame #2 {
                n330 = local write "左"(FALSE ("上")) -> ()
              }
              frame #3 {
                n331 = Wait (ms)(milliseconds to wait=u32 60 ("等待时间（毫秒）")) -> ()  [unwired: 1 out]
              }
            }
          }
          event Timeout {
            w801 = FALSE
            n332 = event-data() -> ()  [unwired: 1 in, 3 out]
            n333 = local write "上"(w801) -> ()
            n334 = local write "右"(w801) -> ()
            n335 = local write "下"(w801) -> ()
            n336 = local write "左"(w801) -> ()
          }
          event "时间到": Value Change {
            n337 = event-data() -> ()  [unwired: 1 in, 1 out]
          }
        }
        n338 = case shown="\"蓝\"" w680 {
          tunnel: w681 -> [_ _ _ _ w716 w724 w732 w742]
          tunnel: w682 -> [_ w707 w710 _ w713 w721 w729 w737]
          tunnel: [w703 w707 w710 w712 w715 w723 w731 w739] -> w677
          tunnel: [w703 0 0 w712 w713 w721 w729 w737] -> w678
          tunnel: ["Game: Read" "Game: Save" "Game: Option" "Game: Exit" w714 w722 w730 w738] -> w676
          frame "读档" {
            w703 = 0
          }
          frame "存档" {
          }
          frame "按错", Default {
          }
          frame "退出" {
            w712 = 0
          }
          frame "黄" {
            n339 = Equal?(x=w716, y=u64 3) -> (x = y?=w718:bool)
            n340 = Increment(x=w713) -> (x+1=w715:i32)
            n341 = case shown="真" w718 {
              tunnel: ["Game: Exit" "Game: Option"] -> w714
              frame False {
              }
              frame True {
              }
            }
          }
          frame "红" {
            n342 = Equal?(x=w724, y=u64 2) -> (x = y?=w726:bool)
            n343 = Increment(x=w721) -> (x+1=w723:i32)
            n344 = case shown="假" w726 {
              tunnel: ["Game: Exit" "Game: Option"] -> w722
              frame False {
              }
              frame True {
              }
            }
          }
          frame "蓝" {
            n345 = Equal?(x=w732, y=u64 1) -> (x = y?=w734:bool)
            n346 = Increment(x=w729) -> (x+1=w731:i32)
            n347 = case shown="真" w734 {
              tunnel: ["Game: Exit" "Game: Option"] -> w730
              frame False {
              }
              frame True {
              }
            }
          }
          frame "绿" {
            n348 = Equal?(x=w742, y=u64 0) -> (x = y?=w741:bool)
            n349 = Increment(x=w737) -> (x+1=w739:i32)
            n350 = case shown="真" w741 {
              tunnel: ["Game: Exit" "Game: Option"] -> w738
              frame False {
              }
              frame True {
              }
            }
          }
        }
        n351 = local read "亮灯次数"() -> (w679:i32)
        n352 = Greater Or Equal?(x=w678, y=w679) -> (x >= y?=w673:bool)
        n353 = local read "时间到"() -> (w675:bool)
        n354 = case shown="假" w675 {
          tunnel: w676 -> [w693 _]
          tunnel: w673 -> [w692 _]
          tunnel: [w691 "Game: Exit"] -> w674
          frame False {
            n355 = case shown="\"Game: Option\", 默认" w693 {
              selector: w693 -> [w695 w699 w700 w701]
              tunnel: w692 -> [w696 _ _ _]
              tunnel: [w694 w699 w700 w701] -> w691
              frame "Game: Option", Default {
                n356 = case shown="真" w696 {
                  tunnel: [w697 "Game: stop counting"] -> w694
                  tunnel: w695 -> [w697 _]
                  frame False {
                  }
                  frame True {
                  }
                }
              }
              frame "Game: Read" {
              }
              frame "Game: Save" {
              }
              frame "Game: Exit" {
              }
            }
          }
          frame True {
          }
        }
        n357 = call <vilib>:"Add State(s) to Queue__JKI_lib_State_Machine.vi"("State(s) in (\"\")"=w690, "State(s) at Back (\"\")"=w674) -> ("States Out"=w689:string)  [unwired: 13 in]
      }
      frame "Game: Exit" {
        # "延时确保倒计时结束"
        # "Template Separator\n(You can make a copy of, or modify, this frame)"
        n358 = local read "难度"() -> (w816:string)
        n359 = local read "分数"() -> (w820:i32)
        n360 = Number To Decimal String(number=w820) -> (decimal integer string=w813:string)  [unwired: 1 in]
        n361 = local write "结束"(TRUE ("停止计时")) -> ()
        n362 = Wait (ms)(milliseconds to wait=u32 5 ("等待时间（毫秒）")) -> ()  [unwired: 1 out]
        n363 = Concatenate Strings("游戏结束！", "\n", "难度：" ("字符串"), w816, "\n", "得分：" ("字符串"), w813) -> (w808:string)
        n364 = Two Button Dialog(message=w808, 1:"结束" ("F按钮名称（“取消”）"), 2:"重新开始" ("T按钮名称（“确定”）")) -> (T button?=w805:bool)
        n365 = case shown="假" w805 {
          tunnel: ["Game: TOP10" ("State(s) at Back (\"\")") "Data: Initialize\nGame: Select_Difficulty" ("State(s) at Back (\"\")")] -> w804
          frame False {
          }
          frame True {
          }
        }
        n366 = call <vilib>:"Add State(s) to Queue__JKI_lib_State_Machine.vi"("State(s) in (\"\")"=w824, "State(s) at Back (\"\")"=w804) -> ("States Out"=w823:string)  [unwired: 13 in]
      }
      frame "Game: stop counting" {
        # "Template Separator\n(You can make a copy of, or modify, this frame)"
        n367 = local read "分数"() -> (w832:i32)
        n368 = Increment(x=w832) -> (x+1=w835:i32)
        n369 = local write "分数"(w835) -> ()
        n370 = local read "亮灯次数"() -> (w831:i32)
        n371 = Increment(x=w831) -> (x+1=w836:i32)
        n372 = local write "亮灯次数"(w836) -> ()
        n373 = local write "是否开始计时？"(FALSE ("是否开始计时？")) -> ()
        n374 = Bundle By Name(cluster=w833, "积分_保存"=w832, "亮灯次数_保存"=w831) -> (w830:T8)
        n375 = Number To Decimal String(number=w835) -> (decimal integer string=w838:string)  [unwired: 1 in]
        n376 = local read "难度"() -> (w840:string)
        n377 = Concatenate Strings(w840, "模式：" ("字符串"), w838, "分" ("字符串")) -> (→"难度：分数":string)
        n378 = Wait (ms)(milliseconds to wait=u32 150 ("等待时间（毫秒）")) -> ()  [unwired: 1 out]
        n379 = call <vilib>:"Add State(s) to Queue__JKI_lib_State_Machine.vi"("State(s) in (\"\")"=w845, "State(s) at Back (\"\")"="Game: Twinkle" ("State(s) at Back (\"\")")) -> ("States Out"=w844:string)  [unwired: 13 in]
      }
      frame "Game: Save" {
        # "Template Separator\n(You can make a copy of, or modify, this frame)"
        n380 = Unbundle By Name(w859) -> ("难度_保存"=w858:string, "亮灯次数_保存"=w856:i32, "超时时间_保存"=w855:i32, "闪烁间隔_保存"=w854:i32, "积分_保存"=w853:i32)
        n381 = case shown="\"简单\"" w858 {
          tunnel: [2 0 1] -> w857
          frame "困难", Default {
          }
          frame "简单" {
          }
          frame "中等" {
          }
        }
        n382 = local write "是否开始计时？"(FALSE ("是否开始计时？")) -> ()
        n383 = Build Array(w857, w856, w855, w854, w853) -> (w852:i32[])
        n384 = Build Array(w848, w852) -> (w849:u64[][])
        n385 = call "文件对话框"("default name"="请选择保存的位置") -> ("selected path"=w850:path)  [unwired: 11 in, 3 out]
        n386 = call-poly <vilib>:"Write Delimited Spreadsheet.vi"("file path (dialog if empty)"=w850, "2D data"=w849) -> ()  [unwired: 12 in, 2 out]
        n387 = call <vilib>:"Add State(s) to Queue__JKI_lib_State_Machine.vi"("State(s) in (\"\")"=w862) -> ("States Out"=w861:string)  [unwired: 14 in]
      }
      frame "Game: TOP10" {
        # "Template Separator\n(You can make a copy of, or modify, this frame)"
        n388 = call <vilib>:"Add State(s) to Queue__JKI_lib_State_Machine.vi"("State(s) in (\"\")"=w871) -> ("States Out"=w870:string)  [unwired: 14 in]
      }
    }
  }
  n389 = disable-structure shown="启用" {
    frame Disabled {
      n390 = while "While循环" {
        shift-right: [w878] -> _
        shift-left: enum16{"倒计时", "初始化"}."初始化" -> [w879]
        stop <- w873 stop-if-true
        # "倒计时"
        n391 = local read "亮灯次数"() -> (w875:i32)
        n392 = Increment(x=w875) -> (x+1=w874:i32)
        n393 = local read "超时时间"() -> (w877:i32)
        n394 = Multiply(x=w877, y=w874) -> (x*y=w876:i32)
        n395 = case shown="\"倒计时\"" w879 {
          tunnel: [enum16{"倒计时", "初始化"}."倒计时" enum16{"倒计时", "初始化"}."倒计时"] -> w878
          tunnel: w876 -> [w881 _]
          tunnel: [w882 FALSE] -> w873
          frame "倒计时" {
            n396 = case shown="假" "是否开始计时？" {
              tunnel: w881 -> [_ w888]
              tunnel: [w885 w887] -> w882
              frame False {
                n397 = local read "结束"() -> (w884:bool)
                n398 = Or(x=w884, y=FALSE) -> (x .or. y?=w885:bool)
              }
              frame True {
                n399 = property on="倒计时" class="Slide (严格)"("Scale.Maximum"=w888) -> ()  [unwired: 2 in, 2 out]
                n400 = for {
                  N: w888 -> [w899]
                  tunnel: [w891] -> w887
                  i -> [w900]
                  stop <- w894 stop-if-true
                  n401 = local read "时间到"() -> (w896:bool)
                  n402 = Subtract(x=w899, y=w900) -> (x-y=w889:i32)
                  "倒计时" <- w889
                  n403 = local read "是否开始计时？"() -> (w897:bool)
                  n404 = Less Or Equal?(x=w889, y=1) -> (x <= y?=w892:bool)
                  n405 = Not(x=w897) -> (.not. x?=w895:bool)
                  n406 = case shown="假" w892 {
                    tunnel: w896 -> [_ w902]
                    frame False {
                    }
                    frame True {
                      n407 = case shown="真" w902 {
                        frame False {
                          (unwired) TRUE ("值(信号)")
                        }
                        frame True {
                          (unwired) FALSE ("值(信号)")
                        }
                      }
                    }
                  }
                  n408 = local read "结束"() -> (w890:bool)
                  n409 = Or(x=w895, y=w892) -> (x .or. y?=w893:bool)
                  n410 = Or(x=w893, y=w890) -> (x .or. y?=w894:bool)
                  n411 = Or(x=w890, y=w892) -> (x .or. y?=w891:bool)
                  n412 = Wait (ms)(milliseconds to wait=u32 1 ("等待时间（毫秒）")) -> ()  [unwired: 1 out]
                }
              }
            }
          }
          frame "初始化", Default {
            n413 = local write "倒计时"(1111111111 ("滑动杆")) -> ()
          }
        }
      }
    }
    frame Enabled {
    }
  }
  n414 = Unbundle By Name(w3) -> ("用户名"=→"字符串":string)
